vi "AFM_Lithography.vi"() -> ()   [LabVIEW 2019]
uses:
  subVIs/Global Variables.vi
  <vilib>/Analysis/Matrix/Datatypes/RealMatrix.ctl
  <vilib>/Analysis/Matrix/NI_Matrix.lvlib
  <userlib>/LevyLab/Relay Box/Typedefs/Resistor--enum.ctl
  <userlib>/LevyLab/Relay Box/Relay-Box.lvclass
  subVIs/AFM API/AFM_Driver_Manager/AFM_Driver_Manager.lvclass
  <vilib>/vision/Image Controls.llb/IMAQ Image.ctl
  <userlib>/LevyLab/Configuration/Configuration.lvclass
  Controls/Configuration.ctl
  Classes/Parse/ParseVectorFile/ParseVectorFile.lvclass
  <vilib>/JKI/JKI SMO/SMO/SMO.lvclass
  Classes/Settings/Setting Database/Setting Database.lvclass
  Classes/Settings/Setting Database/Typedefs/PrivateEvents--Setting Database.Refresh.ctl
  Classes/Parse/Dot/Dot.lvclass
  Classes/Settings/Dot Settings/Dot Settings.lvclass
  Classes/Settings/Path Settings/Path Settings.lvclass
  Classes/Tool/Tool Data/Tool Data/Tool Data.lvclass
  Classes/Settings/Setting Database/Typedefs/PublicEvents--Setting Database.PathsUpdated.ctl
  Classes/Settings/Rectangle Settings/Rectangle Settings.lvclass
  Classes/Settings/Setting Database/Typedefs/PublicEvents--Setting Database.RectanglesUpdated.ctl
  Classes/Settings/Funnel Settings/Funnel Settings.lvclass
  Classes/Settings/Setting Database/Typedefs/PublicEvents--Setting Database.FunnelsUpdated.ctl
  Classes/Settings/Setting Database/Typedefs/PublicEvents--Setting Database.DotsUpdated.ctl
  Classes/Parse/ParsePaths/Path.lvclass
  Classes/Parse/Rectangle/Rectangle.lvclass
  Classes/Parse/Image/SVGImage.lvclass
  Classes/Tool/Tool Data/Tool Data/Typedefs/PrivateEvents--Tool Data.Update Objects.ctl
  <vilib>/Platform/browser.llb/Open URL in Default Browser (string).vi
  Classes/Selector/Selector.lvclass
  <vilib>/Utility/miscctls.llb/LVPositionTypeDef.ctl
  C:/Program Files (x86)/National Instruments/LabVIEW 2019/vi.lib/JKI/JKI SMO/SMO/SMO.lvclass
  Classes/Settings/ObjectSettings/ObjectSettings.lvclass
  C:/Users/Albro/Documents/GitHub/AFM-Lithography/lvsrc/Classes/Settings/ObjectSettings/ObjectSettings.lvclass
  Classes/Tool/Tool Path/Tool Path.lvclass
  C:/Users/Albro/Documents/GitHub/AFM-Lithography/lvsrc/Classes/Tool/Tool Object/Tool Object.lvclass
  Classes/Tool/Tool Funnel/Tool Funnel.lvclass
  C:/Users/Albro/Documents/GitHub/AFM-Lithography/lvsrc/Classes/Tool/Tool Path/Tool Path.lvclass
  Classes/Tool/Tool Rectangle/Tool Rectangle.lvclass
  Classes/Tool/Tool Dot/Tool Dots.lvclass
panel:
  in  "Listbox":i32(listbox)
  out "version":string
  out "Ready?":bool
  out "Estimated Time":string
  in  "Run":bool
  in  "Refresh Button":bool
  in  "Done":bool
  in  "Help":bool
  in  "Abort":bool
  out "Render":T1(plugin-control)
  in  "Settings":T2(tab)
  out "Status":string
  in  "Background Image":path caption="Path"
  in  "Inkscape File (.svg)":path caption="Path"
  in  "Hide Labels?":bool
  in  "Patterns":i32(listbox) caption="Patterns (drag-and-drop reorder)"
  in  "AFM Type":u16(ring) caption="Ring" items=["Asylum"]
  in  "Save Render":bool caption="Save"
  in  "Autosave?":bool
  in  "Autosave Path":path caption="Path"
  in  "Create Overlay":bool
  out "Image Filename":string
  in  "Image Data Range":cluster{dbl, dbl}(slide)={100.0, 0.0} scale=0.0..100.0
  in  "Page":u32 caption="Numeric" max=3
  in  "MCLB":i32(listbox) caption="Multicolumn Listbox 2"
  # "AFM Lithography"
  # "Render"
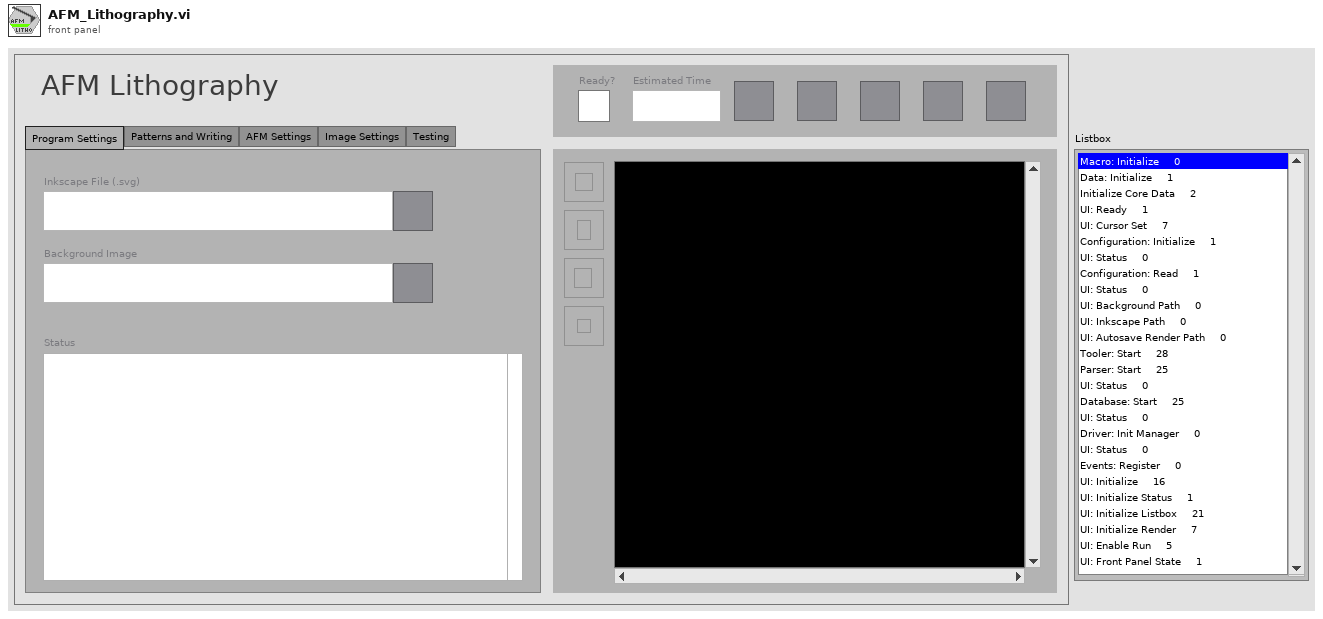
[diagram p1: front panel]
types:
  T1 = typedef "IMAQ Image.ctl" = refnum<image>
  T2 = enum32{"Program Settings", "Patterns and Writing", "AFM Settings", "Image Settings", "Testing"}
  T3 = typedef "LVPositionTypeDef.ctl" = cluster{"Left":i32, "Top":i32}
  T4 = cluster{"Point":T3, "Button":u16, "PlatMods":cluster{"Shift":bool, "Ctrl":bool, "Alt":bool, "Cmd":bool, "Opt":bool}}
  T5 = enum32{"invalid app kind", "Development System", "Run Time System", "Student Edition", "Embedded LabVIEW", "Evaluation", "Custom"}
  T6 = enum32{"Program Settings", "Patterns and Writing", "AFM Settings", "Image Settings"}
  T7 = enum32{"Invalid", "Standard", "Closed", "Hidden", "Minimized", "Maximized"}
  T8 = enum8{"Enabled", "Disabled", "Disabled and Grayed Out"}
  T9 = cluster{"Pattern":string, "Pattern Label":string, "Prompt":string}
  T10 = cluster{"Name":string, "Group":string, "Enabled":bool}
  T11 = typedef "Configuration.ctl" = cluster{"Inkscape Path":path, "Background Path":path, "Autosave Render Path":path, "Autosave Render":bool}
  T12 = typedef "Setting Database.lvclass/PrivateEvents--Setting Database.Refresh.ctl" = cluster{"Paths":string[], "Rectangles":string[], "Funnels":string[], "Dots":string[]}
  T13 = typedef "Tool Data.lvclass/PrivateEvents--Tool Data.Update Objects.ctl" = cluster{"Settings":cluster{"Paths":T14, "Rectangles":T15, "Funnels":T16, "Dots":T17}, "Data":cluster{"Paths":refnum<class "Path.lvclass">[], "Rectangles":refnum<class "Rectangle.lvclass">[], "SVGImage":refnum<class "SVGImage.lvclass">, "Dots":refnum<class "Dot.lvclass">[], "Funnels":refnum<class "Path.lvclass">[]}}
  T14 = typedef "Setting Database.lvclass/PublicEvents--Setting Database.PathsUpdated.ctl" = refnum<class "Path Settings.lvclass">[]
  T15 = typedef "Setting Database.lvclass/PublicEvents--Setting Database.RectanglesUpdated.ctl" = refnum<class "Rectangle Settings.lvclass">[]
  T16 = typedef "Setting Database.lvclass/PublicEvents--Setting Database.FunnelsUpdated.ctl" = refnum<class "Funnel Settings.lvclass">[]
  T17 = typedef "Setting Database.lvclass/PublicEvents--Setting Database.DotsUpdated.ctl" = refnum<class "Dot Settings.lvclass">[]
  T18 = typedef "NI_Matrix.lvlib/RealMatrix.ctl" = dbl[][]
  T19 = typedef "Relay-Box.lvclass/Resistor--enum.ctl" = enum16{"open", "discharge tip", "0 ohms", "100k ohm", "10M ohm", "1G ohm"}
  T20 = cluster{"Core":cluster{"Current VI Reference":refnum<vi>, "Close Panel on Exit?":bool}, "Parsing Data":cluster{"paths":cluster{"Fill Color":string, "Stroke Color":string, "Commands":cluster{"Command Type":string, "Coordinates":cluster{"X":dbl, "Y":dbl}[]}[], "Transformation Matrix 2":T18}[], "funnels":cluster{"Fill Color":string, "Stroke Color":string, "Commands":cluster{"Command Type":string, "Coordinates":cluster{"X":dbl, "Y":dbl}[]}[], "Transformation Matrix 2":T18}[], "rects":cluster{"Fill Color":string, "Stroke Color":string, "Width":dbl, "Height":dbl, "X":dbl, "Y":dbl, "Transformation Matrix":T18}[], "Dots":refnum<class "Dot.lvclass">[]}, "Lithography Data":cluster{"Name":string, "Litho":cluster{"X":dbl, "Y":dbl, "Speed":dbl, "Voltage":dbl}[], "Set Resistance":T19, "Meta":variant}[], "VI Refs":refnum<vi>[], "root path":path, "AFM_Driver_Manager":refnum<class "AFM_Driver_Manager.lvclass">, "IMAQ (Work)":T1, "Background Image":path, "Inkscape File (.svg)":path, "ParseVectorFile":refnum<class "ParseVectorFile.lvclass">, "Database":refnum<class "Setting Database.lvclass">, "Hide Labels":bool, "Autosave?":bool, "Autosave Path":path, "Image Data Range":cluster{dbl, dbl}, "Status":string, "Config":refnum<class "Configuration.lvclass">, "Drag and Drop":cluster{"Start":string[], "End":string[], "Running":string[], "Working":string[]}, "IDs":cluster{"paths":string[], "funnels":string[], "rects":string[], "dots":string[]}, "Tooler":refnum<class "Tool Data.lvclass">, "MCLB":refnum<class "Selector.lvclass">, "Menu Path":string, "Item Names":string[][]}
  T21 = cluster{"Paths":T14, "Rectangles":T15, "Funnels":T16, "Dots":T17}
  T22 = typedef "LVPoint32TypeDef.ctl" = cluster{"Horizontal":i32, "Vertical":i32}
  T23 = cluster{"Shift":bool, "Ctrl":bool, "Alt":bool, "Cmd":bool, "Opt":bool}
  T24 = cluster{"paths":string[], "funnels":string[], "rects":string[], "dots":string[]}
  T25 = cluster{"Start":string[], "End":string[], "Running":string[], "Working":string[]}
  T26 = cluster{"paths":cluster{"Fill Color":string, "Stroke Color":string, "Commands":cluster{"Command Type":string, "Coordinates":cluster{"X":dbl, "Y":dbl}[]}[], "Transformation Matrix 2":T18}[], "funnels":cluster{"Fill Color":string, "Stroke Color":string, "Commands":cluster{"Command Type":string, "Coordinates":cluster{"X":dbl, "Y":dbl}[]}[], "Transformation Matrix 2":T18}[], "rects":cluster{"Fill Color":string, "Stroke Color":string, "Width":dbl, "Height":dbl, "X":dbl, "Y":dbl, "Transformation Matrix":T18}[], "Dots":refnum<class "Dot.lvclass">[]}
  T27 = cluster{"Name":string, "Litho":cluster{"X":dbl, "Y":dbl, "Speed":dbl, "Voltage":dbl}[], "Set Resistance":T19, "Meta":variant}[]
  T28 = cluster{"Current VI Reference":refnum<vi>, "Close Panel on Exit?":bool}
  T29 = typedef "Setting Database.lvclass/PublicEvents--Cluster.ctl" = cluster{"NewActivePath":refnum<user-event>, "PathsUpdated":refnum<user-event>, "RectanglesUpdated":refnum<user-event>, "NewActiveRectangle":refnum<user-event>, "NewActiveFunnel":refnum<user-event>, "FunnelsUpdated":refnum<user-event>, "NewActiveDot":refnum<user-event>, "DotsUpdated":refnum<user-event>}
  T30 = typedef "AFM_Driver_Manager.lvclass/AFM_Driver_Manager.PublicEvents.ctl" = cluster{"Lithography Done":refnum<user-event>}
  T31 = typedef "Image Type" = u32
  T32 = cluster{"Name":string, "Litho":cluster{"X":dbl, "Y":dbl, "Speed":dbl, "Voltage":dbl}[], "Set Resistance":T19, "Meta":variant}
  T33 = cluster{"Name":string, "Group":string, "Enabled":bool}[]
  T34 = typedef "ParseVectorFile.lvclass/PublicEvents--ParseVectorFile.ParsedData.ctl" = cluster{"Paths":refnum<class "Path.lvclass">[], "Rectangles":refnum<class "Rectangle.lvclass">[], "SVGImage":refnum<class "SVGImage.lvclass">, "Dots":refnum<class "Dot.lvclass">[]}
  T35 = cluster{"Paths":refnum<class "Path.lvclass">[], "Rectangles":refnum<class "Rectangle.lvclass">[], "SVGImage":refnum<class "SVGImage.lvclass">, "Dots":refnum<class "Dot.lvclass">[], "Funnels":refnum<class "Path.lvclass">[]}
  T36 = typedef "Tool Data.lvclass/PublicEvents--Tool Data.Objects Updated.ctl" = cluster{"Paths":refnum<class "Tool Path.lvclass">[], "Funnels":refnum<class "Tool Funnel.lvclass">[], "Rectangles":refnum<class "Tool Rectangle.lvclass">[], "Dots":refnum<class "Tool Dots.lvclass">[]}
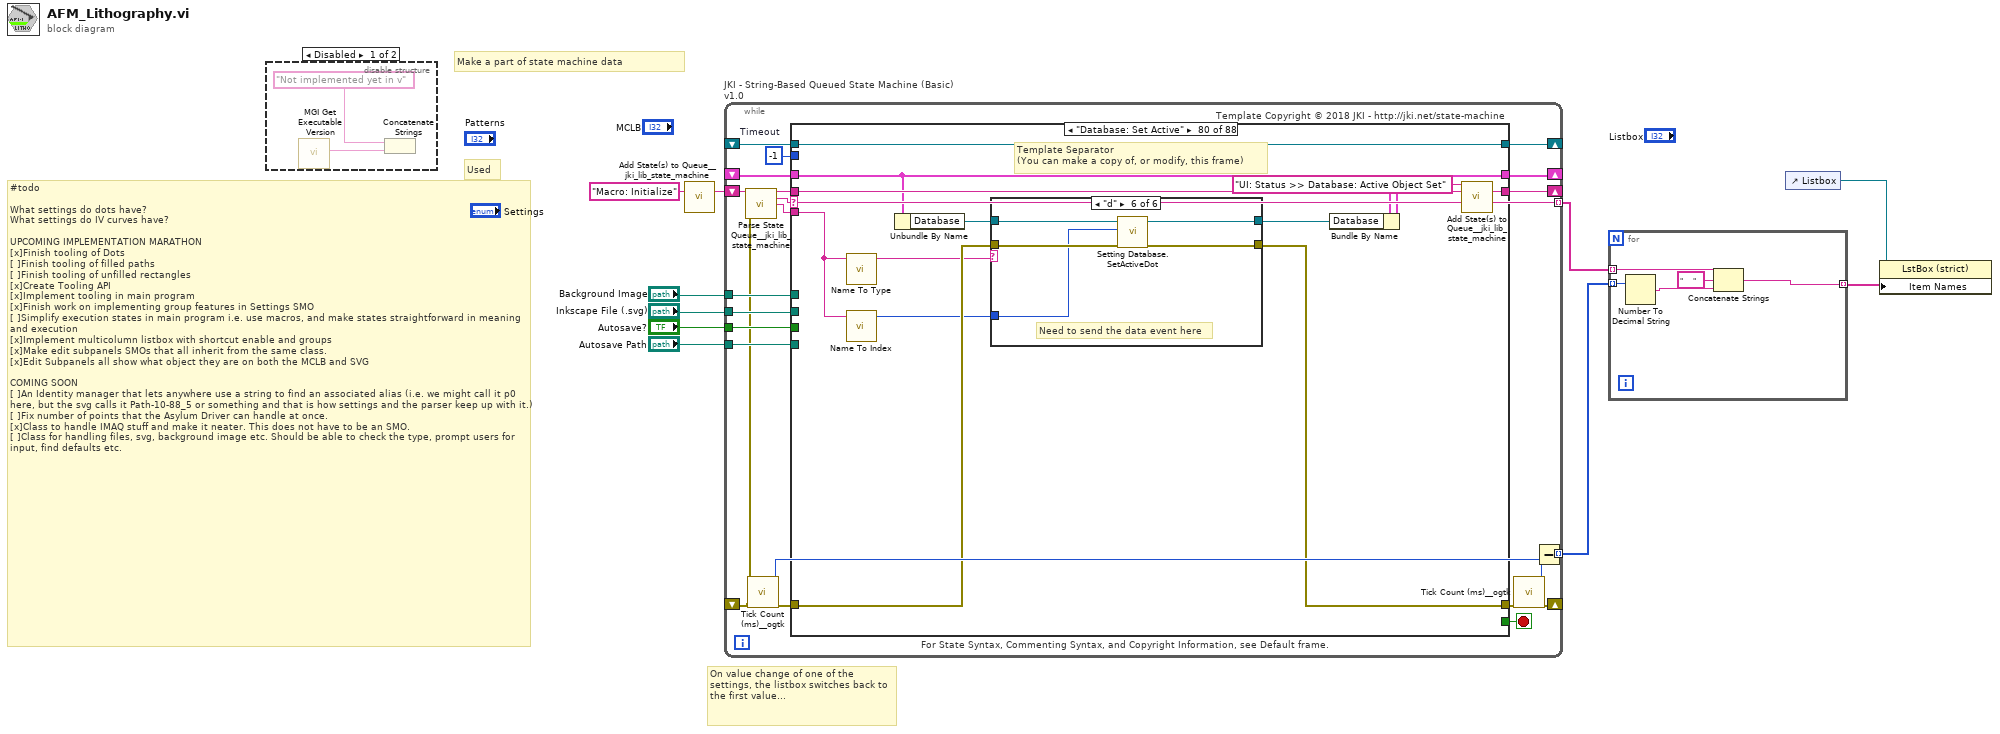
[diagram p0: block diagram]
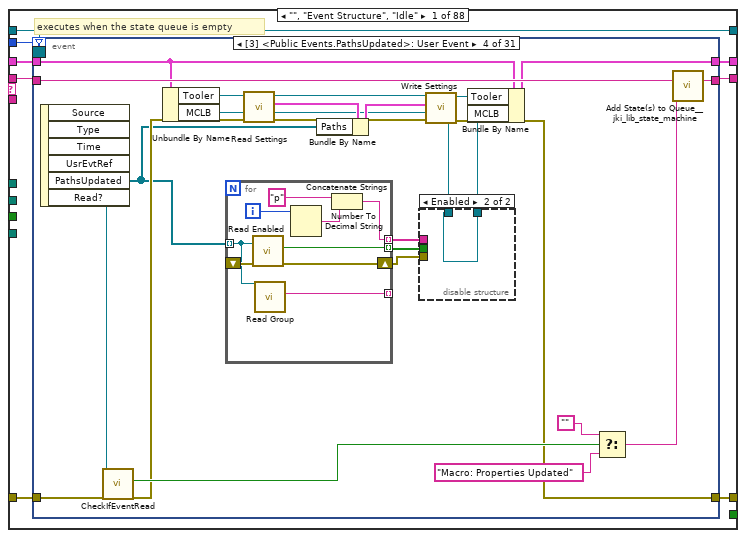
[diagram p3: hidden frame]
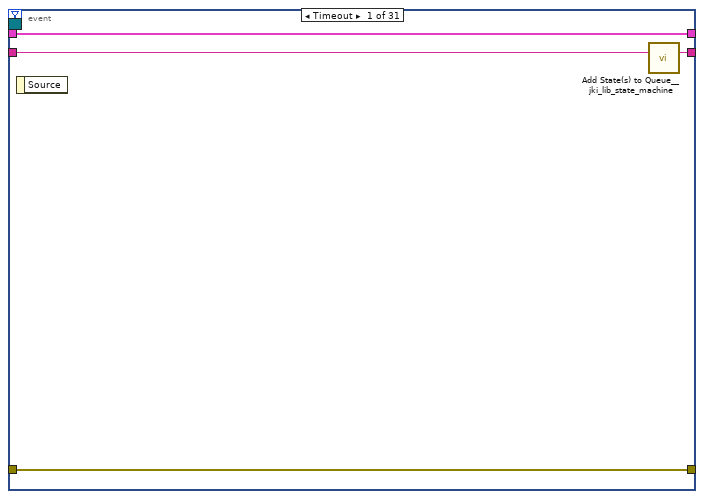
[diagram p4: hidden frame]
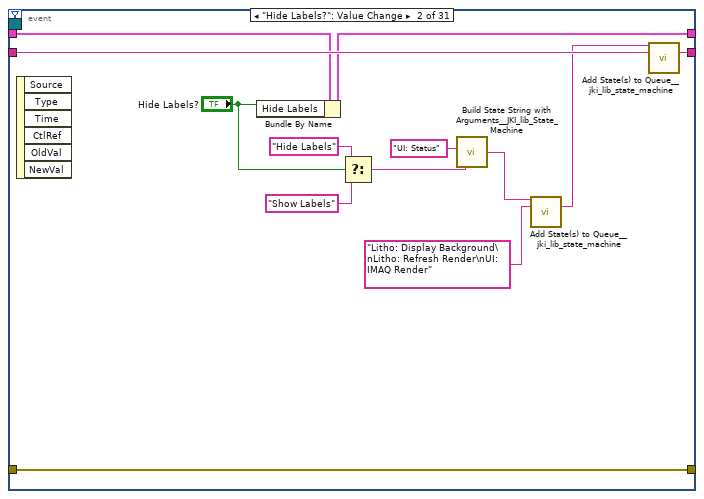
[diagram p5: hidden frame]
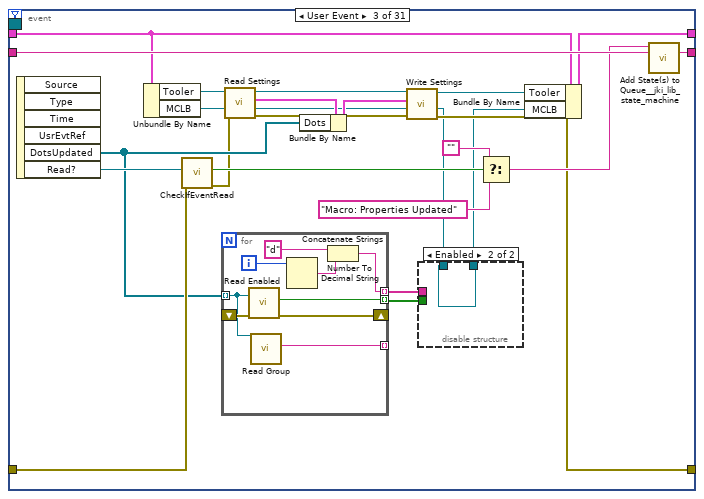
[diagram p6: hidden frame]
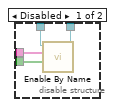
[diagram p7: hidden frame]
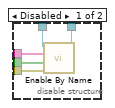
[diagram p8: hidden frame]
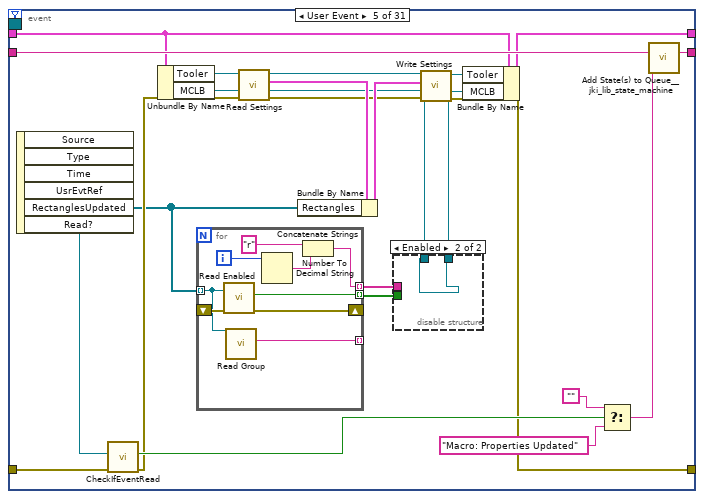
[diagram p9: hidden frame]
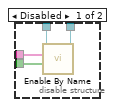
[diagram p10: hidden frame]
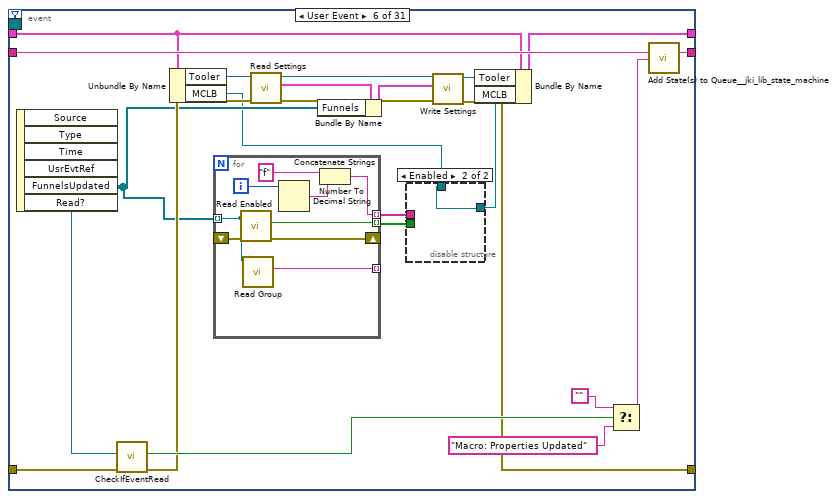
[diagram p11: hidden frame]
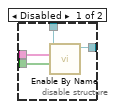
[diagram p12: hidden frame]
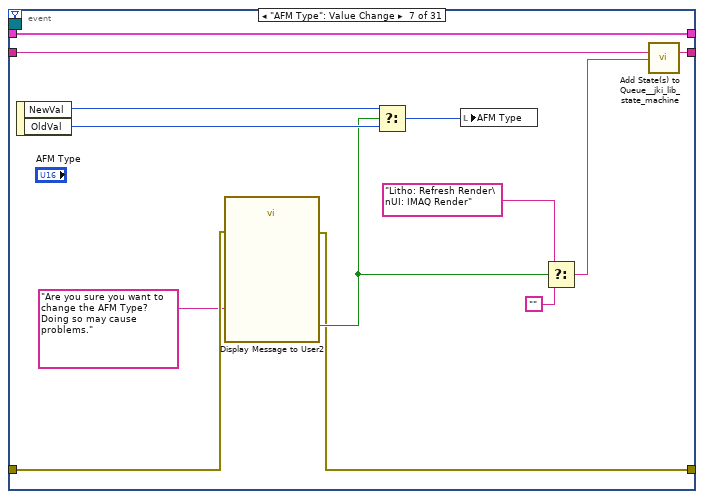
[diagram p13: hidden frame]
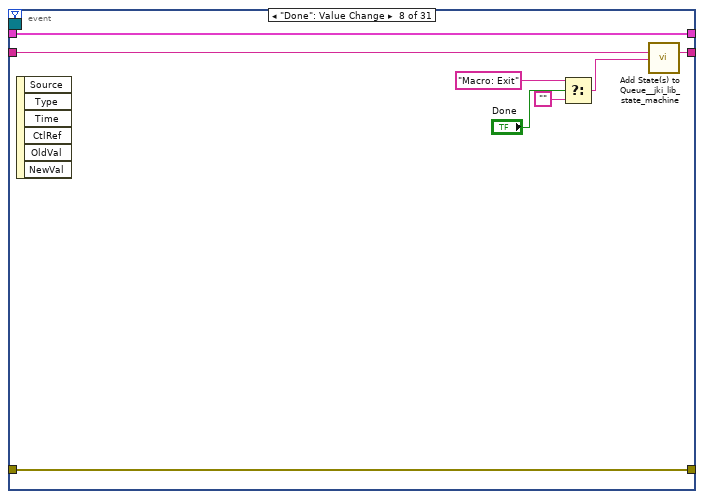
[diagram p14: hidden frame]
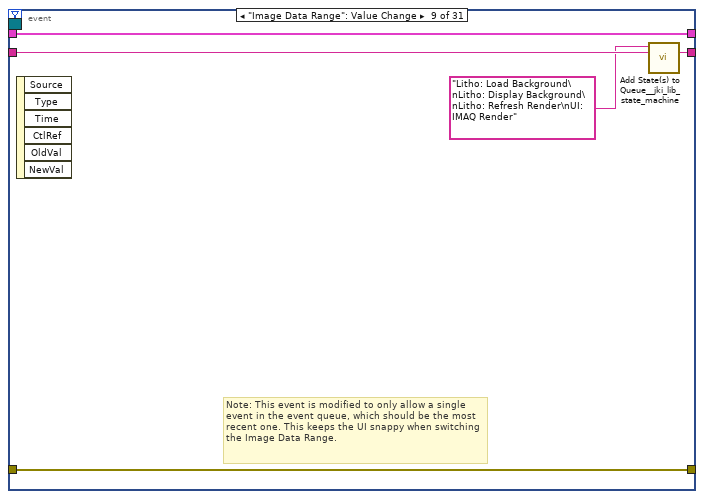
[diagram p15: hidden frame]
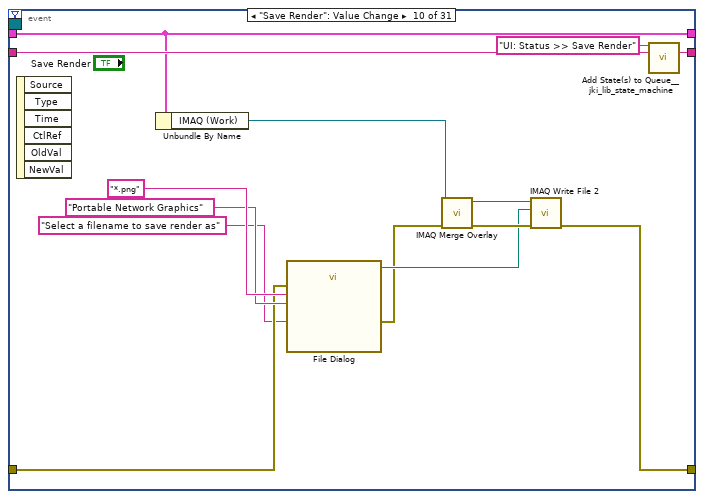
[diagram p16: hidden frame]
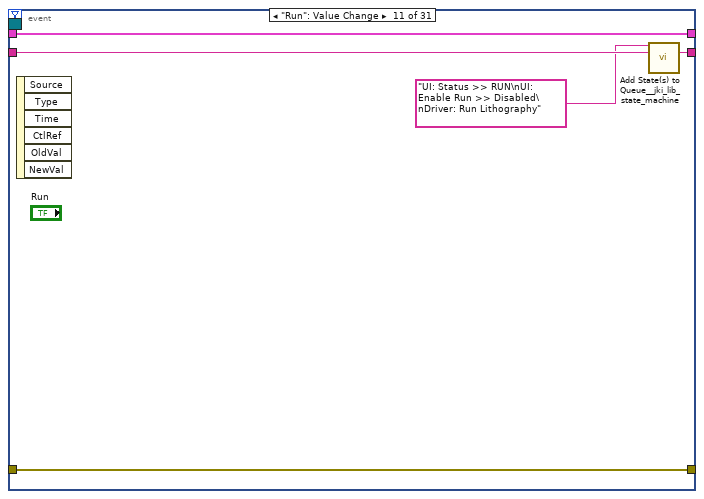
[diagram p17: hidden frame]
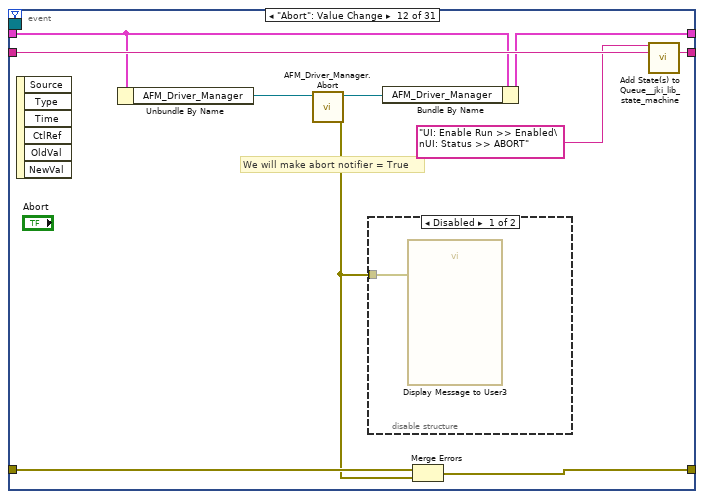
[diagram p18: hidden frame]
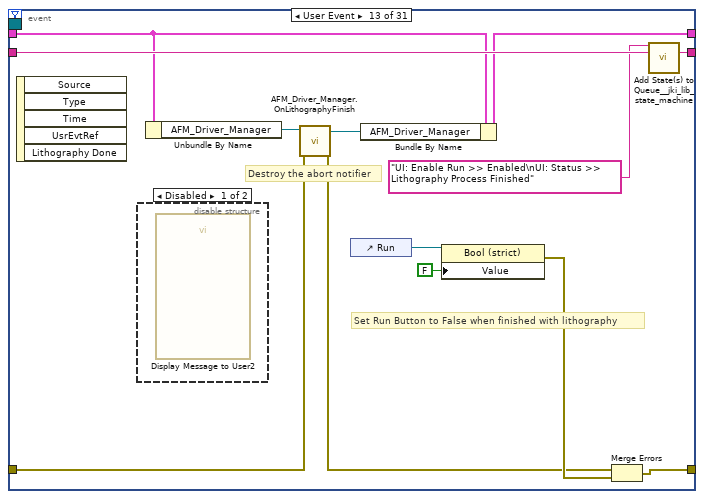
[diagram p20: hidden frame]
diagram:
  # "On value change of one of the settings, the listbox switches back to the first value..."
  # "#todo\n\nWhat settings do dots have?\nWhat settings do IV curves have?\n\nUPCOMING IMPLEMENTATION MARATHON\n[x]Finish tooling of Dots\n[ ]Finish tooling of filled paths\n[ ]Finish tooling of unfilled rectangles\n[x]Create Tooling API\n[x]Implement tooling in main program\n[x]Finish work on implementing group features in Settings SMO\n[ ]Simplify execution states in main program i.e. use macros, and make states straightforward in meaning and execution\n[x]Implement multicolumn listbox with shortcut enable and groups\n[x]Make edit subpanels SMOs that all inherit from the same class.\n[x]Edit Subpanels all show what object they are on both the MCLB and SVG\n\nCOMING SOON\n[ ]An Identity manager that lets anywhere use a string to find an associated alias (i.e. we might call it p0 here, but the svg calls it Path-10-88_5 or something and that is how settings and the parser keep up with it.)\n[ ]Fix number of points that the Asylum Driver can handle at once.\n[x]Class to handle IMAQ stuff and make it neater. This does not have to be an SMO.\n[ ]Class for handling files, svg, background image etc. Should be able to check the type, prompt users for input, find defaults etc."
  # "Used"
  # "Make a part of state machine data"
  n1 = disable-structure shown="Disabled" {
    frame Disabled {
      n2 = call <userlib>:"MGI Get Executable Version.vi"() -> ("Version"=w11:string)  [unwired: 7 in]
      n3 = Concatenate Strings("Not implemented yet in v" ("Status"), w11) -> ()  [unwired: 1 out]
    }
    frame Enabled {
    }
  }
  n4 = call <vilib>:"Add State(s) to Queue__jki_lib_state_machine.vi"("State(s) in (\"\")"="Macro: Initialize") -> ("States Out"=w10:string)  [unwired: 14 in]
  n5 = while "JKI - String-Based Queued State Machine (Basic) v1.0" {
    shift-right: [w32] -> _
    shift-left: _ -> [w31]
    shift-right: [w17] -> _
    shift-left: _ -> [w19]
    shift-right: [w22] -> _
    shift-left: w10 -> [w34]
    shift-right: [w28] -> _
    shift-left: _ -> [w27]
    tunnel: "Background Image" -> [w26]
    tunnel: "Inkscape File (.svg)" -> [w25]
    tunnel: "Autosave?" -> [w24]
    tunnel: "Autosave Path" -> [w23]
    tunnel: [w18] -> w4 mode=indexing
    tunnel: [w13] -> w3 mode=indexing
    stop <- w33 stop-if-true
    w30 = -1  # Timeout
    # "Template Copyright © 2018 JKI - http://jki.net/state-machine"
    # "For State Syntax, Commenting Syntax, and Copyright Information, see Default frame."
    n6 = call <vilib>:"Parse State Queue__jki_lib_state_machine.vi"("State Queue"=w34, "Error In (no error)"=w19) -> ("Remaining States"=w29:string, "Current State"=w18:string, "Arguments"=w21:string)  [unwired: 11 in]
    n7 = call <userlib>:"Tick Count (ms)__ogtk.vi"("error in (no error)"=w19) -> ("error out"=w16:errorcluster, "millisecond timer value"=w14:u32)  [unwired: 9 in]
    n8 = case shown="\"Database: Set Active\"" w18 {
      selector: w18 -> [_ _ w471 _ _ _ _ _ _ _ _ _ _ _ _ _ _ _ _ _ _ _ _ _ _ _ _ _ _ _ _ _ _ _ _ _ _ _ _ _ _ _ _ _ _ _ _ _ _ _ _ _ _ _ _ _ _ _ _ _ _ _ _ _ _ _ _ _ _ _ _ _ _ _ _ _ _ _ _ _ _ _ _ _ _ _ _ _]
      tunnel: w21 -> [_ _ _ _ w498 _ _ _ _ _ _ _ _ _ _ _ _ _ _ w681 w693 w701 w717 w728 _ w771 _ _ _ _ _ _ _ _ _ _ _ _ _ _ _ _ _ _ _ _ _ _ _ _ _ _ _ _ _ _ _ _ _ _ _ _ _ _ _ _ _ w1313 _ _ _ _ _ _ _ _ _ _ w1445 w1455 _ _ _ _ _ _ _ _]
      tunnel: w31 -> [w39 w466 w473 w487 w496 w505 w510 _ w547 w566 w579 w588 w595 w608 w612 w630 w638 w645 w673 w687 w697 w703 w707 w726 w757 w774 w778 w788 w805 w814 w823 w848 w868 w872 w878 w884 w889 w895 w901 w907 w913 w923 w928 w938 w957 w982 w1011 w1021 w1030 w1066 w1076 w1087 w1118 w1126 w1149 w1157 w1171 w1185 w1191 w1214 w1230 w1247 w1265 w1277 w1284 w1288 w1299 w1318 w1329 w1337 w1347 w1357 w1371 w1375 w1408 w1421 w1433 w1439 w1450 w1463 w1510 w1549 w1564 w1576 w1583 w1594 w1605 w1635]
      tunnel: w16 -> [w42 w469 w479 w494 w502 w508 w513 w516 w552 w570 w572 w591 w597 w606 w615 w621 w633 w641 w665 w691 w700 w706 w708 w732 w758 w765 w782 w785 w801 w810 w822 w827 w863 w875 w881 w887 w892 w898 w904 w910 w916 w925 w936 w941 w955 w980 w1014 w1023 w1027 w1056 w1078 w1094 w1113 w1134 w1154 w1156 w1176 w1182 w1196 w1219 w1235 w1239 w1262 w1273 w1286 w1289 w1307 w1315 w1326 w1339 w1344 w1361 w1368 w1380 w1384 w1416 w1427 w1444 w1446 w1460 w1501 w1536 w1555 w1570 w1582 w1588 w1599 w1624]
      tunnel: [w40 w468 w475 w493 w500 w507 w512 w542 w548 w569 w582 w590 w604 w610 w614 w628 w640 w661 w671 w690 w699 w705 w718 w730 w762 w776 w781 w791 w808 w819 w826 w849 w870 w874 w880 w886 w891 w897 w903 w909 w915 w924 w935 w940 w960 w986 w1017 w1022 w1032 w1073 w1077 w1093 w1121 w1133 w1153 w1161 w1175 w1189 w1195 w1218 w1234 w1251 w1269 w1281 w1285 w1296 w1310 w1322 w1333 w1343 w1354 w1365 w1373 w1379 w1413 w1425 w1437 w1443 w1454 w1467 w1514 w1553 w1568 w1580 w1587 w1598 w1609 w1639] -> w22
      tunnel: [_ _ _ _ _ TRUE _ _ _ _ _ _ _ _ _ _ _ _ _ _ _ _ _ _ _ _ _ _ _ _ _ _ _ _ _ _ _ _ _ _ _ _ _ _ _ _ _ _ _ _ _ _ _ _ _ _ _ _ _ _ _ _ _ _ _ _ _ _ _ _ _ _ _ _ _ _ _ _ _ _ _ _ _ _ _ _ _ _] -> w33
      tunnel: [w38 w466 w473 w486 w496 w505 w510 w540 w550 w567 w579 w588 w595 w608 w612 w630 w638 w643 w673 w686 w697 w703 w707 w726 w757 w774 w778 w788 w805 w814 w823 w848 w868 w872 w878 w884 w889 w895 w901 w907 w913 w923 w928 w938 w956 w983 w1015 w1021 w1031 w1067 w1076 w1086 w1118 w1127 w1150 w1158 w1172 w1186 w1192 w1215 w1231 w1248 w1266 w1278 w1284 w1292 w1306 w1320 w1330 w1338 w1349 w1360 w1371 w1376 w1409 w1422 w1434 w1440 w1451 w1464 w1511 w1550 w1565 w1577 w1584 w1595 w1606 w1636] -> w32
      tunnel: w30 -> [w37 _ _ _ _ _ _ _ _ _ _ _ _ _ _ _ _ _ _ _ _ _ _ _ _ _ _ _ _ _ _ _ _ _ _ _ _ _ _ _ _ _ _ _ _ _ _ _ _ _ _ _ _ _ _ _ _ _ _ _ _ _ _ _ _ _ _ _ _ _ _ _ _ _ _ _ _ _ _ _ _ _ _ _ _ _ _ _]
      tunnel: [w41 w469 w480 w494 errorcluster {"status"=FALSE, "code"=0, "source"=""} ("error out") w508 w513 w517 w551 w570 w583 w591 w598 w605 w615 w624 w634 w649 w666 w691 w700 w706 w712 w731 w759 w766 w782 w786 w794 w811 w822 w829 w862 w875 w881 w887 w892 w898 w904 w910 w916 w925 w936 w941 w951 w975 w1007 w1023 w1026 w1055 w1078 w1094 w1112 w1134 w1154 w1156 w1176 w1182 w1196 w1219 w1235 w1238 w1257 w1274 w1286 w1290 w1308 w1316 w1327 w1340 w1345 w1362 w1369 w1380 w1393 w1417 w1428 w1444 w1447 w1461 w1499 w1515 w1557 w1571 w1582 w1589 w1600 w1622] -> w20
      tunnel: w29 -> [w36 w467 w474 w488 w497 w504 w511 w541 w548 w568 w578 w589 w603 w609 w613 w629 w639 w662 w672 w689 w698 w704 w716 w727 w761 w775 w780 w790 w807 w818 w825 w847 w869 w873 w879 w885 w890 w896 w902 w908 w914 w922 w927 w939 w959 w985 w1016 w1020 w1024 w1071 w1075 w1092 w1120 w1132 w1152 w1160 w1174 w1188 w1194 w1217 w1233 w1250 w1268 w1280 w1283 w1295 w1309 w1321 w1332 w1342 w1353 w1364 w1372 w1378 w1412 w1424 w1436 w1442 w1453 w1466 w1513 w1552 w1567 w1579 w1586 w1597 w1608 w1638]
      tunnel: [w35 w465 w470 w482 w495 w503 w509 w539 w544 w563 w575 w587 w602 w607 w611 w627 w637 w652 w667 w688 w696 w702 w715 w725 w760 w773 w779 w789 w806 w817 w824 w846 w864 w871 w877 w882 w888 w894 w900 w906 w912 w918 w926 w937 w958 w984 w1006 w1019 w1029 w1070 w1074 w1091 w1119 w1131 w1151 w1159 w1173 w1187 w1193 w1216 w1232 w1249 w1267 w1279 w1282 w1294 w1301 w1314 w1324 w1335 w1348 w1358 w1367 w1377 w1411 w1423 w1435 w1441 w1452 w1465 w1512 w1551 w1566 w1578 w1585 w1596 w1607 w1637] -> w28
      tunnel: w27 -> [w35 w465 w470 w482 w495 w503 w509 w539 w544 w563 w575 w587 _ w607 w611 w627 w637 w652 w667 w688 w696 w702 w715 w725 w760 w773 w779 w789 w806 w817 w824 w846 w864 w871 w877 w882 w888 w894 w900 w906 w912 w918 w926 w937 w958 w984 w1006 w1019 w1029 w1070 w1074 w1091 w1119 w1131 w1151 w1159 w1173 w1187 w1193 w1216 w1232 w1249 w1267 w1279 w1282 w1294 w1301 w1314 w1324 w1335 w1348 w1358 w1367 w1377 w1411 w1423 w1435 w1441 w1452 w1465 w1512 w1551 w1566 w1578 w1585 w1596 w1607 w1637]
      tunnel: w26 -> [_ _ _ _ _ _ _ w538 _ _ _ _ _ _ _ _ _ _ _ _ _ _ _ _ _ _ _ _ _ _ _ _ _ _ _ _ _ _ _ _ _ _ _ _ _ _ _ _ _ _ _ _ _ _ _ _ _ _ _ _ _ _ _ _ _ _ _ _ _ _ _ _ _ _ _ _ _ _ _ _ _ _ _ _ _ _ _ _]
      tunnel: w25 -> [_ _ _ _ _ _ _ w537 _ _ _ _ _ _ _ _ _ _ _ _ _ _ _ _ _ _ _ _ _ _ _ _ _ _ _ _ _ _ _ _ _ _ _ _ _ _ _ _ _ _ _ _ _ _ _ _ _ _ _ _ _ _ _ _ _ _ _ _ _ _ _ _ _ _ _ _ _ _ _ _ _ _ _ _ _ _ _ _]
      tunnel: w24 -> [_ _ _ _ _ _ _ w527 _ _ _ _ _ _ _ _ _ _ _ _ _ _ _ _ _ _ _ _ _ _ _ _ _ _ _ _ _ _ _ _ _ _ _ _ _ _ _ _ _ _ _ _ _ _ _ _ _ _ _ _ _ _ _ _ _ _ _ _ _ _ _ _ _ _ _ _ _ _ _ _ _ _ _ _ _ _ _ _]
      tunnel: w23 -> [_ _ _ _ _ _ _ w526 _ _ _ _ _ _ _ _ _ _ _ _ _ _ _ _ _ _ _ _ _ _ _ _ _ _ _ _ _ _ _ _ _ _ _ _ _ _ _ _ _ _ _ _ _ _ _ _ _ _ _ _ _ _ _ _ _ _ _ _ _ _ _ _ _ _ _ _ _ _ _ _ _ _ _ _ _ _ _ _]
      frame "", "Event Structure", "Idle" {
        # "executes when the state queue is empty"
        n9 = event shown="[3] <Public Events.PathsUpdated>: User Event" {
          selector: w35 -> [_ _ _ _ _ _ _ _ _ _ _ _ _ _ _ _ _ _ _ _ _ _ _ _ _ _ _ _ _ _ _]
          dyn-events: _ -> [_ _ _ _ _ _ _ _ _ _ _ _ _ _ _ _ _ _ _ _ _ _ _ _ _ _ _ _ _ _ _]
          timeout: w37 -> [_ _ _ _ _ _ _ _ _ _ _ _ _ _ _ _ _ _ _ _ _ _ _ _ _ _ _ _ _ _ _]
          tunnel: w36 -> [w46 w59 w82 w120 w158 w195 w220 w227 w232 w248 w251 w263 w277 w280 w295 w306 w318 w325 w330 w335 w340 w344 w355 w366 w383 w401 w432 w436 w446 w457 w463]
          tunnel: [w45 w58 w81 w119 w157 w194 w221 w228 w233 w249 w252 w264 w278 w281 w294 w305 w317 w324 w329 w334 w339 w343 w354 w365 w382 w400 w431 w435 w445 w456 w462] -> w40
          tunnel: w39 -> [w44 w55 w66 w106 w144 w181 w222 w229 w234 w247 w253 w258 w270 w283 w292 w303 w316 w321 w327 w333 w341 w345 w351 w361 w380 w396 w428 w437 w442 w453 w461]
          tunnel: w42 -> [w43 w57 w76 w118 w154 w191 w212 w230 w235 w239 w254 w260 w271 w285 w296 w307 w319 w326 w331 w336 w337 w346 w347 w357 w384 w390 w433 w438 w440 w458 w464]
          tunnel: [w44 w56 w71 w104 w141 w178 w222 w229 w234 w247 w253 w259 w273 w283 w293 w304 w309 w322 w327 w333 w341 w345 w352 w362 w381 w395 w429 w437 w443 w454 w461] -> w38
          tunnel: [w43 w57 w67 w98 w142 w179 w211 w230 w235 w243 w254 w261 w267 w284 w296 w307 w319 w326 w331 w336 w337 w346 w348 w358 w384 w391 w433 w438 w439 w458 w464] -> w41
          event Timeout {
            n10 = event-data() -> ()  [unwired: 1 in, 1 out]
            n11 = call <vilib>:"Add State(s) to Queue__jki_lib_state_machine.vi"("State(s) in (\"\")"=w46) -> ("States Out"=w45:string)  [unwired: 14 in]
          }
          event "Hide Labels?": Value Change {
            n12 = event-data() -> ()  [unwired: 1 in, 6 out]
            n13 = Bundle By Name(cluster=w55, "Hide Labels"="Hide Labels?") -> (w56:T20)
            n14 = Select(t="Hide Labels" ("State(s) in Front (\"\")"), s="Hide Labels?", f="Show Labels" ("State(s) in Front (\"\")")) -> (s? t:f=w50:string)
            n15 = call <vilib>:"Build State String with Arguments__JKI_lib_State_Machine.vi"("Arguments (\"\")"=w50, "State"="UI: Status") -> ("State with Arguments"=w49:string)  [unwired: 4 in]
            n16 = call <vilib>:"Add State(s) to Queue__jki_lib_state_machine.vi"("State(s) in Front (\"\")"=w49, "State(s) in (\"\")"="Litho: Display Background\nLitho: Refresh Render\nUI: IMAQ Render") -> ("States Out"=w53:string)  [unwired: 13 in]
            n17 = call <vilib>:"Add State(s) to Queue__jki_lib_state_machine.vi"("State(s) in Front (\"\")"=w53, "State(s) in (\"\")"=w59) -> ("States Out"=w58:string)  [unwired: 13 in]
          }
          event User Event {
            n18 = event-data() -> ("DotsUpdated"=w65:T17, "Read?"=w80:refnum<notifier>)  [unwired: 1 in, 4 out]
            n19 = Unbundle By Name(w66) -> ("Tooler"=w74:refnum<class "Tool Data.lvclass">, "MCLB"=w62:refnum<class "Selector.lvclass">)
            n20 = call "CheckIfEventRead.vi"("error in (no error)"=w76, "Read?"=w80) -> ("error out"=w60:errorcluster, "Read"=w75:bool)  [unwired: 8 in]
            n21 = for {
              tunnel: w65 -> [w89] mode=indexing
              tunnel: [w96] -> w63 mode=indexing
              tunnel: [w92] -> w64 mode=indexing
              shift-right: [w91] -> _
              shift-left: _ -> [w90]
              tunnel: [w88] -> _ mode=indexing
              i -> [w94]
              n22 = call "Read Enabled.vi"("error in (no error)"=w90, "ObjectSettings in"=w89) -> ("error out"=w91:errorcluster, "Enabled"=w96:bool)  [unwired: 7 in, 1 out]
              n23 = call-dynamic "Read Group.vi"("ObjectSettings in"=w89) -> ("Group"=w88:string)  [unwired: 8 in, 2 out]
              n24 = Number To Decimal String(number=w94) -> (decimal integer string=w93:string)  [unwired: 1 in]
              n25 = Concatenate Strings("d" ("string"), w93) -> (w92:string)
            }
            n26 = call-dynamic "Read Settings.vi"("error in (no error)"=w60, "Tool Data in"=w74) -> ("error out"=w68:errorcluster, "Settings"=w70:T21, "Tool Data out"=w73:refnum<class "Tool Data.lvclass">)  [unwired: 7 in]
            n27 = Bundle By Name(cluster=w70, "Dots"=w65) -> (w69:T21)
            n28 = call-dynamic "Write Settings.vi"("error in (no error)"=w68, "Settings"=w69, "Tool Data in"=w73) -> ("error out"=w67:errorcluster, "Tool Data out"=w72:refnum<class "Tool Data.lvclass">)  [unwired: 7 in]
            n29 = disable-structure shown="Enabled" {
              disable-tunnel: w64 -> [w86 _]
              disable-tunnel: w63 -> [w85 _]
              disable-tunnel: w62 -> [w84 w87]
              disable-tunnel: [w83 w87] -> w61
              frame Disabled {
                n30 = call-dynamic "Enable By Name.vi"("Enable Items"=w85, "Names"=w86, "Selector in"=w84) -> ("Selector out"=w83:refnum<class "Selector.lvclass">)  [unwired: 7 in, 1 out]
              }
              frame Enabled {
              }
            }
            n31 = Select(t="", s=w75, f="Macro: Properties Updated") -> (s? t:f=w77:string)
            n32 = Bundle By Name(cluster=w66, "Tooler"=w72, "MCLB"=w61) -> (w71:T20)
            n33 = call <vilib>:"Add State(s) to Queue__jki_lib_state_machine.vi"("State(s) in Front (\"\")"=w77, "State(s) in (\"\")"=w82) -> ("States Out"=w81:string)  [unwired: 13 in]
          }
          event User Event {
            n34 = event-data() -> ("PathsUpdated"=w101:T14, "Read?"=w117:refnum<notifier>)  [unwired: 1 in, 4 out]
            n35 = call "CheckIfEventRead.vi"("error in (no error)"=w118, "Read?"=w117) -> ("error out"=w105:errorcluster, "Read"=w113:bool)  [unwired: 8 in]
            n36 = Unbundle By Name(w106) -> ("Tooler"=w112:refnum<class "Tool Data.lvclass">, "MCLB"=w100:refnum<class "Selector.lvclass">)
            n37 = for {
              tunnel: w101 -> [w128] mode=indexing
              tunnel: [w135] -> w102 mode=indexing
              tunnel: [w131] -> w103 mode=indexing
              shift-right: [w130] -> w97
              shift-left: _ -> [w129]
              tunnel: [w127] -> _ mode=indexing
              i -> [w133]
              n38 = call "Read Enabled.vi"("error in (no error)"=w129, "ObjectSettings in"=w128) -> ("error out"=w130:errorcluster, "Enabled"=w135:bool)  [unwired: 7 in, 1 out]
              n39 = call-dynamic "Read Group.vi"("ObjectSettings in"=w128) -> ("Group"=w127:string)  [unwired: 8 in, 2 out]
              n40 = Number To Decimal String(number=w133) -> (decimal integer string=w132:string)  [unwired: 1 in]
              n41 = Concatenate Strings("p" ("string"), w132) -> (w131:string)
            }
            n42 = call-dynamic "Read Settings.vi"("error in (no error)"=w105, "Tool Data in"=w112) -> ("error out"=w107:errorcluster, "Settings"=w109:T21, "Tool Data out"=w111:refnum<class "Tool Data.lvclass">)  [unwired: 7 in]
            n43 = Bundle By Name(cluster=w109, "Paths"=w101) -> (w108:T21)
            n44 = disable-structure shown="Enabled" {
              disable-tunnel: w103 -> [w125 _]
              disable-tunnel: w102 -> [w124 _]
              disable-tunnel: w100 -> [w123 w126]
              disable-tunnel: [w122 w126] -> w99
              disable-tunnel: w97 -> [w121 _]
              frame Disabled {
                n45 = call-dynamic "Enable By Name.vi"("error in (no error)"=w121, "Enable Items"=w124, "Names"=w125, "Selector in"=w123) -> ("Selector out"=w122:refnum<class "Selector.lvclass">)  [unwired: 6 in, 1 out]
              }
              frame Enabled {
              }
            }
            n46 = call-dynamic "Write Settings.vi"("error in (no error)"=w107, "Settings"=w108, "Tool Data in"=w111) -> ("error out"=w98:errorcluster, "Tool Data out"=w110:refnum<class "Tool Data.lvclass">)  [unwired: 7 in]
            n47 = Bundle By Name(cluster=w106, "Tooler"=w110, "MCLB"=w99) -> (w104:T20)
            n48 = Select(t="", s=w113, f="Macro: Properties Updated") -> (s? t:f=w114:string)
            n49 = call <vilib>:"Add State(s) to Queue__jki_lib_state_machine.vi"("State(s) in (\"\")"=w120, "State(s) at Back (\"\")"=w114) -> ("States Out"=w119:string)  [unwired: 13 in]
          }
          event User Event {
            n50 = event-data() -> ("RectanglesUpdated"=w138:T15, "Read?"=w153:refnum<notifier>)  [unwired: 1 in, 4 out]
            n51 = call "CheckIfEventRead.vi"("error in (no error)"=w154, "Read?"=w153) -> ("error out"=w143:errorcluster, "Read"=w151:bool)  [unwired: 8 in]
            n52 = Unbundle By Name(w144) -> ("Tooler"=w150:refnum<class "Tool Data.lvclass">, "MCLB"=w137:refnum<class "Selector.lvclass">)
            n53 = for {
              tunnel: w138 -> [w165] mode=indexing
              tunnel: [w172] -> w139 mode=indexing
              tunnel: [w168] -> w140 mode=indexing
              shift-right: [w167] -> _
              shift-left: _ -> [w166]
              tunnel: [w164] -> _ mode=indexing
              i -> [w170]
              n54 = call "Read Enabled.vi"("error in (no error)"=w166, "ObjectSettings in"=w165) -> ("error out"=w167:errorcluster, "Enabled"=w172:bool)  [unwired: 7 in, 1 out]
              n55 = call-dynamic "Read Group.vi"("ObjectSettings in"=w165) -> ("Group"=w164:string)  [unwired: 8 in, 2 out]
              n56 = Number To Decimal String(number=w170) -> (decimal integer string=w169:string)  [unwired: 1 in]
              n57 = Concatenate Strings("r" ("string"), w169) -> (w168:string)
            }
            n58 = call-dynamic "Read Settings.vi"("error in (no error)"=w143, "Tool Data in"=w150) -> ("error out"=w145:errorcluster, "Settings"=w147:T21, "Tool Data out"=w149:refnum<class "Tool Data.lvclass">)  [unwired: 7 in]
            n59 = Bundle By Name(cluster=w147, "Rectangles"=w138) -> (w146:T21)
            n60 = disable-structure shown="Enabled" {
              disable-tunnel: w140 -> [w162 _]
              disable-tunnel: w139 -> [w161 _]
              disable-tunnel: w137 -> [w160 w163]
              disable-tunnel: [w159 w163] -> w136
              frame Disabled {
                n61 = call-dynamic "Enable By Name.vi"("Enable Items"=w161, "Names"=w162, "Selector in"=w160) -> ("Selector out"=w159:refnum<class "Selector.lvclass">)  [unwired: 7 in, 1 out]
              }
              frame Enabled {
              }
            }
            n62 = call-dynamic "Write Settings.vi"("error in (no error)"=w145, "Settings"=w146, "Tool Data in"=w149) -> ("error out"=w142:errorcluster, "Tool Data out"=w148:refnum<class "Tool Data.lvclass">)  [unwired: 7 in]
            n63 = Bundle By Name(cluster=w144, "Tooler"=w148, "MCLB"=w136) -> (w141:T20)
            n64 = Select(t="", s=w151, f="Macro: Properties Updated") -> (s? t:f=w152:string)
            n65 = call <vilib>:"Add State(s) to Queue__jki_lib_state_machine.vi"("State(s) in (\"\")"=w158, "State(s) at Back (\"\")"=w152) -> ("States Out"=w157:string)  [unwired: 13 in]
          }
          event User Event {
            n66 = event-data() -> ("FunnelsUpdated"=w175:T16, "Read?"=w190:refnum<notifier>)  [unwired: 1 in, 4 out]
            n67 = call "CheckIfEventRead.vi"("error in (no error)"=w191, "Read?"=w190) -> ("error out"=w180:errorcluster, "Read"=w188:bool)  [unwired: 8 in]
            n68 = Unbundle By Name(w181) -> ("Tooler"=w187:refnum<class "Tool Data.lvclass">, "MCLB"=w173:refnum<class "Selector.lvclass">)
            n69 = for {
              tunnel: [w201] -> _ mode=indexing
              tunnel: [w209] -> w176 mode=indexing
              tunnel: [w205] -> w177 mode=indexing
              shift-right: [w204] -> _
              shift-left: _ -> [w203]
              tunnel: [w202] -> _ mode=indexing
              tunnel: w175 -> [w201] mode=indexing
              i -> [w207]
              n70 = call "Read Enabled.vi"("error in (no error)"=w203, "ObjectSettings in"=w201) -> ("error out"=w204:errorcluster, "Enabled"=w209:bool)  [unwired: 7 in, 1 out]
              n71 = call-dynamic "Read Group.vi"("ObjectSettings in"=w201) -> ("Group"=w202:string)  [unwired: 8 in, 2 out]
              n72 = Number To Decimal String(number=w207) -> (decimal integer string=w206:string)  [unwired: 1 in]
              n73 = Concatenate Strings("f" ("string"), w206) -> (w205:string)
            }
            n74 = call-dynamic "Read Settings.vi"("error in (no error)"=w180, "Tool Data in"=w187) -> ("error out"=w182:errorcluster, "Settings"=w184:T21, "Tool Data out"=w186:refnum<class "Tool Data.lvclass">)  [unwired: 7 in]
            n75 = Bundle By Name(cluster=w184, "Funnels"=w175) -> (w183:T21)
            n76 = disable-structure shown="Enabled" {
              disable-tunnel: w177 -> [w199 _]
              disable-tunnel: w176 -> [w198 _]
              disable-tunnel: [w197 w200] -> w174
              disable-tunnel: w173 -> [w196 w200]
              frame Disabled {
                n77 = call-dynamic "Enable By Name.vi"("Enable Items"=w198, "Names"=w199, "Selector in"=w196) -> ("Selector out"=w197:refnum<class "Selector.lvclass">)  [unwired: 7 in, 1 out]
              }
              frame Enabled {
              }
            }
            n78 = call-dynamic "Write Settings.vi"("error in (no error)"=w182, "Settings"=w183, "Tool Data in"=w186) -> ("error out"=w179:errorcluster, "Tool Data out"=w185:refnum<class "Tool Data.lvclass">)  [unwired: 7 in]
            n79 = Bundle By Name(cluster=w181, "Tooler"=w185, "MCLB"=w174) -> (w178:T20)
            n80 = Select(t="", s=w188, f="Macro: Properties Updated") -> (s? t:f=w189:string)
            n81 = call <vilib>:"Add State(s) to Queue__jki_lib_state_machine.vi"("State(s) in (\"\")"=w195, "State(s) at Back (\"\")"=w189) -> ("States Out"=w194:string)  [unwired: 13 in]
          }
          event "AFM Type": Value Change {
            n82 = event-data() -> ("NewVal"=w216:u16, "OldVal"=w215:u16)  [unwired: 1 in]
            n83 = call "Display Message to User2"("error in (no error)"=w212, "Message"="Are you sure you want to change the AFM Type? Doing so may cause problems.") -> ("error out"=w211:errorcluster, "OK?"=w213:bool)  [unwired: 8 in]
            n84 = Select(t=w216, s=w213, f=w215) -> (s? t:f=w214:u16)
            n85 = local write "AFM Type"(w214) -> ()
            n86 = Select(t="Litho: Refresh Render\nUI: IMAQ Render" ("State(s) at Back (\"\")"), s=w213, f="" ("Empty String Constant")) -> (s? t:f=w217:string)
            n87 = call <vilib>:"Add State(s) to Queue__jki_lib_state_machine.vi"("State(s) in (\"\")"=w220, "State(s) at Back (\"\")"=w217) -> ("States Out"=w221:string)  [unwired: 13 in]
          }
          event "Done": Value Change {
            n88 = event-data() -> ()  [unwired: 1 in, 6 out]
            n89 = Select(t="Macro: Exit", s="Done", f="" ("Empty String Constant")) -> (s? t:f=w223:string)
            n90 = call <vilib>:"Add State(s) to Queue__jki_lib_state_machine.vi"("State(s) in (\"\")"=w227, "State(s) at Back (\"\")"=w223) -> ("States Out"=w228:string)  [unwired: 13 in]
          }
          event "Image Data Range": Value Change {
            # "Note: This event is modified to only allow a single event in the event queue, which should be the most recent one. This keeps the UI snappy when switching the Image Data Range."
            n91 = event-data() -> ()  [unwired: 1 in, 6 out]
            n92 = call <vilib>:"Add State(s) to Queue__jki_lib_state_machine.vi"("State(s) in Front (\"\")"="Litho: Load Background\nLitho: Display Background\nLitho: Refresh Render\nUI: IMAQ Render", "State(s) in (\"\")"=w232) -> ("States Out"=w233:string)  [unwired: 13 in]
          }
          event "Save Render": Value Change {
            n93 = event-data() -> ()  [unwired: 1 in, 6 out]
            n94 = Unbundle By Name(w247) -> ("IMAQ (Work)"=w245:T1)
            n95 = call "File Dialog"("prompt"="Select a filename to save render as", "error in"=w239, "pattern (all files)"="*.png", "pattern label"="Portable Network Graphics") -> ("selected path"=w242:path, "error out"=w237:errorcluster)  [unwired: 8 in, 2 out]
            n96 = call "IMAQ Merge Overlay"("error in (no error)"=w237, "Image Src"=w245) -> ("error out"=w246:errorcluster, "Image Dst Out"=w244:T1)  [unwired: 8 in]
            n97 = call-poly "IMAQ Write File 2"("error in (no error)"=w246, "File Path"=w242, "Image"=w244) -> ("error out"=w243:errorcluster)  [unwired: 7 in, 1 out]
            n98 = call <vilib>:"Add State(s) to Queue__jki_lib_state_machine.vi"("State(s) in Front (\"\")"="UI: Status >> Save Render" ("State(s) in Front (\"\")"), "State(s) in (\"\")"=w248) -> ("States Out"=w249:string)  [unwired: 13 in]
          }
          event "Run": Value Change {
            n99 = event-data() -> ()  [unwired: 1 in, 6 out]
            n100 = call <vilib>:"Add State(s) to Queue__jki_lib_state_machine.vi"("State(s) in Front (\"\")"="UI: Status >> RUN\nUI: Enable Run >> Disabled\nDriver: Run Lithography", "State(s) in (\"\")"=w251) -> ("States Out"=w252:string)  [unwired: 13 in]
          }
          event "Abort": Value Change {
            # "We will make abort notifier = True"
            n101 = event-data() -> ()  [unwired: 1 in, 6 out]
            n102 = Unbundle By Name(w258) -> ("AFM_Driver_Manager"=w262:refnum<class "AFM_Driver_Manager.lvclass">)
            n103 = call "AFM_Driver_Manager.Abort.vi"("AFM_Driver_Manager in"=w262) -> ("error out"=w256:errorcluster, "AFM_Driver_Manager out"=w257:refnum<class "AFM_Driver_Manager.lvclass">)  [unwired: 9 in]
            n104 = disable-structure "Diagram Disable Structure" shown="Disabled" {
              disable-tunnel: w256 -> [w265 _]
              frame Disabled {
                n105 = call "Display Message to User3"("error in (no error)"=w265) -> ()  [unwired: 9 in, 2 out]
              }
              frame Enabled {
              }
            }
            n106 = Bundle By Name(cluster=w258, "AFM_Driver_Manager"=w257) -> (w259:T20)
            n107 = Merge Errors(w260, w256) -> (w261:errorcluster)
            n108 = call <vilib>:"Add State(s) to Queue__jki_lib_state_machine.vi"("State(s) in Front (\"\")"="UI: Enable Run >> Enabled\nUI: Status >> ABORT", "State(s) in (\"\")"=w263) -> ("States Out"=w264:string)  [unwired: 13 in]
          }
          event User Event {
            # "Destroy the abort notifier"
            # "Set Run Button to False when finished with lithography"
            n109 = event-data() -> ()  [unwired: 1 in, 5 out]
            n110 = disable-structure "Diagram Disable Structure" shown="Disabled" {
              frame Disabled {
                n111 = call "Display Message to User2"() -> ()  [unwired: 10 in, 2 out]
              }
              frame Enabled {
              }
            }
            n112 = Unbundle By Name(w270) -> ("AFM_Driver_Manager"=w274:refnum<class "AFM_Driver_Manager.lvclass">)
            n113 = call "AFM_Driver_Manager.OnLithographyFinish.vi"("error in (no error)"=w271, "AFM_Driver_Manager in"=w274) -> ("error out"=w268:errorcluster, "AFM_Driver_Manager out"=w272:refnum<class "AFM_Driver_Manager.lvclass">)  [unwired: 8 in]
            n114 = control-ref of="Run"() -> (w276:refnum<vi>)
            n115 = Bundle By Name(cluster=w270, "AFM_Driver_Manager"=w272) -> (w273:T20)
            n116 = property on="Property Node" class="Bool (strict)"(reference=w276, "Value"=FALSE) -> (error out=w269:errorcluster)  [unwired: 1 in, 1 out]
            n117 = Merge Errors(w268, w269) -> (w267:errorcluster)
            n118 = call <vilib>:"Add State(s) to Queue__jki_lib_state_machine.vi"("State(s) in Front (\"\")"="UI: Enable Run >> Enabled\nUI: Status >> Lithography Process Finished" ("State(s) in Front (\"\")"), "State(s) in (\"\")"=w277) -> ("States Out"=w278:string)  [unwired: 13 in]
          }
          event "Help": Value Change {
            n119 = event-data() -> ()  [unwired: 1 in, 6 out]
            n120 = call-poly <vilib>:"Open URL in Default Browser.vi"("error in (no error)"=w285, "URL"="https://github.com/levylabpitt/AFM-Lithography") -> ("error out"=w284:errorcluster)  [unwired: 4 in, 1 out]
            n121 = call <vilib>:"Add State(s) to Queue__jki_lib_state_machine.vi"("State(s) in Front (\"\")"="UI: Status >> HELP" ("State(s) in Front (\"\")"), "State(s) in (\"\")"=w280) -> ("States Out"=w281:string)  [unwired: 13 in]
          }
          event "Inkscape File (.svg)": Value Change {
            n122 = event-data() -> ("NewVal"=w291:path)  [unwired: 1 in, 5 out]
            n123 = Bundle By Name(cluster=w292, "Inkscape File (.svg)"=w291) -> (w293:T20)
            n124 = call <vilib>:"Build State String with Arguments__JKI_lib_State_Machine.vi"("Arguments (\"\")"="Inkscape File Changed" ("Arguments (\"\")"), "State"="UI: Status") -> ("State with Arguments"=w290:string)  [unwired: 4 in]
            n125 = call <vilib>:"Add State(s) to Queue__jki_lib_state_machine.vi"("State(s) in Front (\"\")"=w290, "State(s) in (\"\")"="UI: Ready >> FALSE\nMacro: Refresh\n//Macro: Send Driver\nConfiguration: Write\nUI: Ready >> TRUE") -> ("States Out"=w286:string)  [unwired: 13 in]
            n126 = call <vilib>:"Add State(s) to Queue__jki_lib_state_machine.vi"("State(s) in Front (\"\")"=w286, "State(s) in (\"\")"=w295) -> ("States Out"=w294:string)  [unwired: 13 in]
          }
          event "Autosave?": Value Change {
            n127 = event-data() -> ("NewVal"=w302:bool)  [unwired: 1 in, 5 out]
            n128 = Bundle By Name(cluster=w303, "Autosave?"=w302) -> (w304:T20)
            n129 = Select(t="UI: Autosave Render", s=w302, f="") -> (s? t:f=w301:string)
            n130 = call <vilib>:"Add State(s) to Queue__jki_lib_state_machine.vi"("State(s) in Front (\"\")"="Configuration: Write" ("State(s) in Front (\"\")"), "State(s) in (\"\")"=w301) -> ("States Out"=w297:string)  [unwired: 13 in]
            n131 = call <vilib>:"Add State(s) to Queue__jki_lib_state_machine.vi"("State(s) in Front (\"\")"=w297, "State(s) in (\"\")"=w306) -> ("States Out"=w305:string)  [unwired: 13 in]
          }
          event "Autosave Path": Value Change {
            n132 = event-data() -> ("NewVal"=w315:path)  [unwired: 1 in, 5 out]
            n133 = Bundle By Name(cluster=w316, "Autosave Path"=w315) -> (w309:T20)
            n134 = Unbundle By Name(w309) -> ("Autosave?"=w308:bool)
            n135 = Select(t="UI: Autosave Render", s=w308, f="") -> (s? t:f=w314:string)
            n136 = call <vilib>:"Add State(s) to Queue__jki_lib_state_machine.vi"("State(s) in Front (\"\")"="Configuration: Write" ("State(s) in Front (\"\")"), "State(s) in (\"\")"=w314) -> ("States Out"=w310:string)  [unwired: 13 in]
            n137 = call <vilib>:"Add State(s) to Queue__jki_lib_state_machine.vi"("State(s) in Front (\"\")"=w310, "State(s) in (\"\")"=w318) -> ("States Out"=w317:string)  [unwired: 13 in]
          }
          event "Background Image": Value Change {
            n138 = event-data() -> ("NewVal"=w320:path)  [unwired: 1 in, 5 out]
            n139 = Bundle By Name(cluster=w321, "Background Image"=w320) -> (w322:T20)
            n140 = call <vilib>:"Add State(s) to Queue__jki_lib_state_machine.vi"("State(s) in Front (\"\")"="UI: Status >> Background Image Changed\nUI: Ready >> FALSE\nLitho: Load Background\nLitho: Display Background\nLitho: Refresh Render\nUI: IMAQ Render\nDriver: Background Image\nUI: Ready >> TRUE\nConfiguration: Write", "State(s) in (\"\")"=w325) -> ("States Out"=w324:string)  [unwired: 13 in]
          }
          event "Create Overlay": Value Change {
            n141 = event-data() -> ()  [unwired: 1 in, 6 out]
            n142 = call <vilib>:"Add State(s) to Queue__jki_lib_state_machine.vi"("State(s) in Front (\"\")"="UI: Status >> Create Overlay\nUI: Ready >> FALSE\nUI: Overlay\nUI: Ready >> TRUE", "State(s) in (\"\")"=w330) -> ("States Out"=w329:string)  [unwired: 13 in]
          }
          event "Page": Value Change {
            n143 = event-data() -> ()  [unwired: 1 in, 6 out]
            n144 = call <vilib>:"Add State(s) to Queue__jki_lib_state_machine.vi"("State(s) in Front (\"\")"="UI: Status >> Image Page Changed\nUI: Ready >> FALSE\nLitho: Load Background\nLitho: Display Background\nLitho: Refresh Render\nUI: IMAQ Render\nUI: Ready >> TRUE", "State(s) in (\"\")"=w335) -> ("States Out"=w334:string)  [unwired: 13 in]
          }
          event "Refresh Button": Value Change {
            n145 = event-data() -> ()  [unwired: 1 in, 6 out]
            n146 = call <vilib>:"Add State(s) to Queue__jki_lib_state_machine.vi"("State(s) in Front (\"\")"="UI: Status >> REFRESH\nUI: Ready >> FALSE\nMacro: Refresh\nMacro: Send Driver\nUI: Ready >> TRUE", "State(s) in (\"\")"=w340) -> ("States Out"=w339:string)  [unwired: 13 in]
          }
          event "Patterns": Value Change {
            n147 = event-data() -> ()  [unwired: 1 in, 6 out]
            n148 = call <vilib>:"Add State(s) to Queue__jki_lib_state_machine.vi"("State(s) in (\"\")"=w344, "State(s) at Back (\"\")"="UI: Status >> New Active Object Selected\nUI: Update Subpanel\nLitho: Order Data\nDriver: Litho Data" ("State(s) at Back (\"\")")) -> ("States Out"=w343:string)  [unwired: 13 in]
          }
          event "MCLB": Value Change {
            n149 = event-data() -> ("NewVal"=w349:i32)  [unwired: 1 in, 5 out]
            n150 = Unbundle By Name(w351) -> ("MCLB"=w353:refnum<class "Selector.lvclass">)
            n151 = call-dynamic "Write Value.vi"("error in (no error)"=w347, "Value"=w349, "Selector in"=w353) -> ("error out"=w348:errorcluster, "Selector out"=w350:refnum<class "Selector.lvclass">)  [unwired: 7 in]
            n152 = Bundle By Name(cluster=w351, "MCLB"=w350) -> (w352:T20)
            n153 = call <vilib>:"Add State(s) to Queue__jki_lib_state_machine.vi"("State(s) in (\"\")"=w355) -> ("States Out"=w354:string)  [unwired: 14 in]
          }
          event "MCLB": Shortcut Menu Activation? {
            n154 = event-data() -> ("MenuRef"=w364:refnum<k9>, "Coords"=w363:T22)  [unwired: 1 in, 5 out]
            n155 = Unbundle By Name(w361) -> ("MCLB"=w360:refnum<class "Selector.lvclass">)
            n156 = disable-structure shown="Enabled" {
              disable-tunnel: w364 -> [w372 _]
              disable-tunnel: w363 -> [w371 _]
              disable-tunnel: w360 -> [w370 w374]
              disable-tunnel: [w369 w374] -> w359
              disable-tunnel: [w368 w373] -> w358
              disable-tunnel: w357 -> [w367 w373]
              frame Disabled {
                n157 = call-dynamic "Populate Menu Activation.vi"("error in (no error)"=w367, "Point32"=w371, "MenuRef"=w372, "Selector in"=w370) -> ("error out"=w368:errorcluster, "Selector out"=w369:refnum<class "Selector.lvclass">)  [unwired: 6 in]
              }
              frame Enabled {
              }
            }
            n158 = Bundle By Name(cluster=w361, "MCLB"=w359) -> (w362:T20)
            n159 = event-data("Discard?"=FALSE) -> ()  [unwired: 1 in, 1 out]
            n160 = call <vilib>:"Add State(s) to Queue__jki_lib_state_machine.vi"("State(s) in (\"\")"=w366) -> ("States Out"=w365:string)  [unwired: 14 in]
          }
          event "MCLB": Shortcut Menu Selection (User) {
            n161 = event-data() -> ("ItemPath"=w376:string)  [unwired: 1 in, 7 out]
            n162 = Bundle By Name(cluster=w380, "Menu Path"=w376) -> (w381:T20)
            n163 = Match Pattern(string=w376, regular expression="\\:") -> (before substring=w377:string)  [unwired: 1 in, 3 out]
            n164 = call <vilib>:"Build State String with Arguments__JKI_lib_State_Machine.vi"("Arguments (\"\")"=w377, "State"="MCLB: SCM Selection") -> ("State with Arguments"=w375:string)  [unwired: 4 in]
            n165 = call <vilib>:"Add State(s) to Queue__jki_lib_state_machine.vi"("State(s) in Front (\"\")"=w375, "State(s) in (\"\")"=w383) -> ("States Out"=w382:string)  [unwired: 13 in]
          }
          event "MCLB": Mouse Down? {
            n166 = event-data() -> ("Coords"=w393:T22, "Button"=w392:u16, "PlatMods"=w388:T23)  [unwired: 1 in, 5 out]
            n167 = Unbundle By Name(w396) -> ("MCLB"=w398:refnum<class "Selector.lvclass">)
            n168 = disable-structure shown="Enabled" {
              disable-tunnel: w398 -> [w411 w425]
              disable-tunnel: [w410 w425] -> w397
              disable-tunnel: w393 -> [w409 _]
              disable-tunnel: w392 -> [w408 _]
              disable-tunnel: [w407 w424] -> w391
              disable-tunnel: w390 -> [w406 w424]
              disable-tunnel: [w405 _] -> w389
              disable-tunnel: w388 -> [w404 _]
              disable-tunnel: [w403 _] -> w387
              disable-tunnel: ["Database: Update Enable" _] -> w386
              frame Disabled {
                n169 = Bundle By Name(cluster=T4 {"Point"={"Left"=0, "Top"=0}, "Button"=0, "PlatMods"={"Shift"=FALSE, "Ctrl"=FALSE, "Alt"=FALSE, "Cmd"=FALSE, "Opt"=FALSE}} ("Event Data"), "Point"=w409, "Button"=w408, "PlatMods"=w404) -> (w412:T4)
                n170 = call-dynamic "Handle Mouse Down.vi"("error in (no error)"=w406, "Event Data"=w412, "Selector in"=w411) -> ("error out"=w414:errorcluster, "Enable Change"=w405:bool, "Selector out"=w413:refnum<class "Selector.lvclass">)  [unwired: 6 in]
                n171 = case shown="True" w405 {
                  tunnel: w413 -> [w418 w423]
                  tunnel: w414 -> [w417 w422]
                  tunnel: [w417 w421] -> w407
                  tunnel: [w418 w420] -> w410
                  tunnel: ["" ("Name") w419] -> w403
                  frame False {
                  }
                  frame True {
                    n172 = call "Change Active Enable Symbol.vi"("error in (no error)"=w422, "Selector in"=w423) -> ("error out"=w421:errorcluster, "Name"=w419:string, "Selector out"=w420:refnum<class "Selector.lvclass">)  [unwired: 7 in]
                  }
                }
              }
              frame Enabled {
              }
            }
            n173 = Bundle By Name(cluster=w396, "MCLB"=w397) -> (w395:T20)
            n174 = call <vilib>:"Build State String with Arguments__JKI_lib_State_Machine.vi"("Arguments (\"\")"=w387, "State"=w386) -> ("State with Arguments"=w385:string)  [unwired: 4 in]
            n175 = Select(t=w385, s=w389, f="") -> (s? t:f=w394:string)
            n176 = event-data("Discard?"=w389) -> ()  [unwired: 4 in, 1 out]
            n177 = call <vilib>:"Add State(s) to Queue__jki_lib_state_machine.vi"("State(s) in Front (\"\")"=w394, "State(s) in (\"\")"=w401) -> ("States Out"=w400:string)  [unwired: 13 in]
          }
          event "MCLB": Drag Ended {
            n178 = event-data() -> ("CtlRef"=w430:refnum<vi>)  [unwired: 1 in, 4 out]
            n179 = property class="MCListbox (strict)"(reference=w430) -> ("ItemNames"=w427:string[][])  [unwired: 1 in, 2 out]
            n180 = Bundle By Name(cluster=w428, "Item Names"=w427) -> (w429:T20)
            n181 = call <vilib>:"Add State(s) to Queue__jki_lib_state_machine.vi"("State(s) in Front (\"\")"="MCLB: Reorder", "State(s) in (\"\")"=w432) -> ("States Out"=w431:string)  [unwired: 13 in]
          }
          event "MCLB": Drag Starting {
            n182 = event-data() -> ()  [unwired: 1 in, 10 out]
            n183 = call <vilib>:"Add State(s) to Queue__jki_lib_state_machine.vi"("State(s) in (\"\")"=w436, "State(s) at Back (\"\")"="UI: Status >> New Active Object Selected\nUI: Update Subpanel\nLitho: Order Data\nDriver: Litho Data" ("State(s) at Back (\"\")")) -> ("States Out"=w435:string)  [unwired: 13 in]
          }
          event "Patterns": Drag Starting {
            n184 = event-data() -> ("CtlRef"=w444:refnum<vi>)  [unwired: 1 in, 9 out]
            n185 = property class="LstBox (strict)"(reference=w444, error in=w440) -> (error out=w439:errorcluster, "Item Names"=w441:string[])  [unwired: 1 out]
            n186 = Bundle By Name(cluster=w442, "Drag and Drop.Start"=w441) -> (w443:T20)
            n187 = call <vilib>:"Add State(s) to Queue__jki_lib_state_machine.vi"("State(s) in (\"\")"=w446) -> ("States Out"=w445:string)  [unwired: 14 in]
          }
          event "Patterns": Drag Ended {
            n188 = event-data() -> ("CtlRef"=w455:refnum<vi>)  [unwired: 1 in, 4 out]
            n189 = property class="LstBox (strict)"(reference=w455) -> ("Item Names"=w448:string[])  [unwired: 1 in, 2 out]
            n190 = Unbundle By Name(w453) -> ("Drag and Drop.Start"=w452:string[])
            n191 = Equal?(x=w452, y=w448) -> (x = y?=w451:bool)
            n192 = Select(t="" ("State(s) in Front (\"\")"), s=w451, f="//Listbox: Compare Values\nListbox: Reorder Data\n//Litho: Order Data\nDriver: Litho Data\nLitho: Refresh Render") -> (s? t:f=w447:string)
            n193 = Bundle By Name(cluster=w453, "Drag and Drop.Working"=w448, "Drag and Drop.Running"=w448) -> (w454:T20)
            n194 = call <vilib>:"Add State(s) to Queue__jki_lib_state_machine.vi"("State(s) in Front (\"\")"=w447, "State(s) in (\"\")"=w457) -> ("States Out"=w456:string)  [unwired: 13 in]
          }
          event Panel Close? {
            # "Discard the event because we'll close the front panel ourselves in Macro: Exit"
            # "Close Panel button (pressed) Event\n(this executes Macro: Exit to terminate the VI)"
            n195 = event-data() -> ()  [unwired: 1 in, 1 out]
            n196 = event-data ("Event Filter Node")("Discard?"=TRUE) -> ()  [unwired: 1 in, 1 out]
            n197 = call <vilib>:"Add State(s) to Queue__jki_lib_state_machine.vi"("State(s) in Front (\"\")"="Macro: Exit", "State(s) in (\"\")"=w463) -> ("States Out"=w462:string)  [unwired: 13 in]
          }
        }
      }
      frame "---------- Core ----------" {
        # "Do not put any code in this frame.\n(it is a separator no-op)"
        n198 = call <vilib>:"Add State(s) to Queue__jki_lib_state_machine.vi"("State(s) in (\"\")"=w467) -> ("States Out"=w468:string)  [unwired: 14 in]
      }
      frame Default {
        w477 = 42 items=["No error", "Argument error", "Memory is full", "Out of zone", "End of file", "File already open", "Generic file I/O error", "File not found", "File permission error", "Disk is full", "Duplicate path", "Too many files open", "System feature not enabled", "Resource file not found", "Cannot add resource", "Resource not found", "Image not found", "Image memory error", "Pen does not exist", "Config type invalid", "Config token not found", "Config parse error", "Config memory error", "Bad external code format", "Bad external code offset", "External code not present", "Null window", "Destroy window error", "Null menu", "Print aborted", "Bad print record", "Print driver error", "Windows error during printing", "Memory error during printing", "Print dialog error", "Generic print error", "Invalid device refnum", "Device not found", "Device parameter error", "Device unit error", "Cannot open device", "Device call aborted", "Generic error", "Cancelled by user", "Object ID too low", "Object ID too high", "Object not in heap", "Unknown heap", "Unknown object (invalid DefProc)", "Unknown object (DefProc not in table)", "Message out of range", "Invalid (null) method", "Unknown message", "Manager call not supported", "Bad address", "Network operation in progress", "Network operation timed out", "Connection is busy", "Network attribute not supported", "Network error", "Address in use", "System out of memory", "Connection aborted", "Connection refused", "Not connected", "Already connected", "Connection closed", "Initialization error (interapplication manager)", "Bad occurrence", "Wait on unbound occurrence handler", "Occurrence queue overflow", "Datalog type conflict", "Unused", "Unrecognized type (interapplication manager)", "Memory corrupt", "Failed to make temporary DLL", "Old CIN version", "Drag socket not found", "Failed to load drop-object", "Failed to register OLE object", "Failed to release OLE object", "Format specifier type mismatch", "Unknown format specifier", "Too few format specifiers", "Too many format specifiers", "Scan failed", "Newer CIN version", "Error converting to variant", "Runtime menu error", "Password tampered", "Variant attribute not found", "Incompatible variant data type", "Event data is not available", "Event Store is not present", "Occurrence is not found", "Event Queue is not created", "Event info is not available", "Refnum passed is NULL", "Error retrieving Class GUID", "Error retrieving CoClass GUID", "Error retrieving TypeLib GUID.", "Bad built application magic bytes.", "Specific driver is different from the specific driver associated with the Logical Name.", "There is no session opened to the class driver.", "Max Error", "MAX - Error with config objects", "MAX - Error loading configuration", "MAX - Group not supported"]
        # "State Syntax:\nStateCategory: State >> Argument\nLine Terminator: Line feed\nExample:\nUI: Help >> About\n\nWhere \"UI\" is the state category\nWhere \"Help\" is the state\nWhere \"About\" is the argument\nOther Examples:\nApp Data: Initialize\nUI: Initialize\nHelp >> About\n\nCommenting:\nTo add a comment use \"//\" or \"#\" and all text to the right will be ignored\nCommenting Example:\nUI: Initialize // This initializes the UI\n# This whole line is a comment\n// Another comment line"
        # "For instructions on how to use the JKI State Machine, examples and video tutorials, visit:\nhttp://jki.net/state-machine/\n\nJKI State Machine™\nhttp://jki.net/state-machine/\nCopyright (C) 2005-2018, JKI <info@jki.net>\nALL RIGHTS RESERVED"
        # "Handle mistyped state name (developer tool)"
        # "Current State"
        # "Do not delete, rename, or modify this frame.\n(this is used to capture unhandled states and typos)"
        n199 = Format Into String(format string="Software Exception: Unhandled State \"%s\"." ("message"), error in=w479, w471) -> (resulting string=w476:string, error out=w481:errorcluster)  [unwired: 1 in]
        n200 = call <vilib>:"Error Cluster From Error Code.vi"("show call chain? (False)"=TRUE, "error in (no error)"=w481, "error message (\"\")"=w476, "error code (0)"=w477) -> ("error out"=w480:errorcluster)  [unwired: 5 in]
        n201 = call <vilib>:"Add State(s) to Queue__jki_lib_state_machine.vi"("State(s) in (\"\")"=w474) -> ("States Out"=w475:string)  [unwired: 14 in]
      }
      frame "Initialize Core Data" {
        # "Do not delete, rename, or modify this frame.\n(this is used to determine panel behavior on exit)"
        # "originally closed?"
        # "exe?"
        # "If panel starts closed or is an EXE, then close it when we exit"
        n202 = property on="Property Node" class="VI"() -> ("Front Panel.Open"=w492:bool)  [unwired: 2 in, 2 out]
        n203 = property on="Property Node" class="App"() -> ("App.Kind"=w491:T5)  [unwired: 2 in, 2 out]
        n204 = control-ref of="Current VI Reference"() -> (w489:refnum<vi>)
        n205 = Not(x=w492) -> (.not. x?=w485:bool)
        n206 = Equal?(x=w491, y=T5."Run Time System" ("Application:Kind")) -> (x = y?=w484:bool)
        n207 = Or(x=w485, y=w484) -> (x .or. y?=w490:bool)
        n208 = Bundle By Name(cluster=w487, "Core.Current VI Reference"=w489, "Core.Close Panel on Exit?"=w490) -> (w486:T20)
        n209 = call <vilib>:"Add State(s) to Queue__jki_lib_state_machine.vi"("State(s) in (\"\")"=w488) -> ("States Out"=w493:string)  [unwired: 14 in]
      }
      frame "Error Handler" {
        # "Unhandled Error -- Display it"
        # "Handle any errors here.\nYou can also output any states to clean-up after errors occur"
        # "Clear error"
        n210 = call <vilib>:"General Error Handler.vi"("[error source] (\" \")"=w498, "error in (no error)"=w502) -> ()  [unwired: 9 in, 5 out]
        n211 = call <vilib>:"Add State(s) to Queue__jki_lib_state_machine.vi"("State(s) in Front (\"\")"="/* Post Error States", "State(s) in (\"\")"=w497) -> ("States Out"=w500:string)  [unwired: 13 in]
      }
      frame "Exit" {
        # "Do not put any code in this frame.\n(No errors that occur here will be handled.)"
        n212 = call <vilib>:"Add State(s) to Queue__jki_lib_state_machine.vi"("State(s) in (\"\")"=w504) -> ("States Out"=w507:string)  [unwired: 14 in]
      }
      frame "---------- Data ----------" {
        # "Do not put any code in this frame.\n(It is a separator no-op. You can make a copy of this frame to create a new Data frame)"
        n213 = call <vilib>:"Add State(s) to Queue__jki_lib_state_machine.vi"("State(s) in (\"\")"=w511) -> ("States Out"=w512:string)  [unwired: 14 in]
      }
      frame "Data: Initialize" {
        w514 = string[][] []  # Item Names
        w515 = ""  # Menu Path
        w521 = refnum<class "Tool Data.lvclass"> refnum  # Tooler
        w522 = T24 {"paths"=[], "funnels"=[], "rects"=[], "dots"=[]}  # IDs
        w535 = T25 {"Start"=[], "End"=[], "Running"=[], "Working"=[]}  # Drag and Drop
        w536 = refnum<class "Configuration.lvclass"> refnum  # Config
        w520 = ""  # Status
        w523 = cluster{dbl, dbl} {100.0, 0.0}  # Image Data Range
        w524 = FALSE  # Hide Labels
        w525 = refnum<class "Setting Database.lvclass"> refnum  # Database
        w528 = refnum<class "ParseVectorFile.lvclass"> refnum  # ParseVectorFile
        w529 = T1 refnum  # IMAQ (Work)
        w530 = refnum<class "AFM_Driver_Manager.lvclass"> refnum  # AFM_Driver_Manager
        w531 = path ""  # root path
        w534 = T26 {"paths"=[], "funnels"=[], "rects"=[], "Dots"=[]}  # Parsing Data
        w532 = refnum<vi>[] []  # VI Refs
        w533 = T27 []  # Lithography Data
        w543 = T28 {"Current VI Reference"=refnum, "Close Panel on Exit?"=FALSE}  # Core
        # "Initialize the shift-register data, here.\n(data names are defined by what you wire into the bundle function)"
        n214 = control-ref of="MCLB"() -> (w518:refnum<vi>)
        n215 = call "Constructor.vi"("error in (no error)"=w516, "Reference"=w518) -> ("error out"=w517:errorcluster, "MCLB"=w519:refnum<class "Selector.lvclass">)  [unwired: 8 in]
        n216 = Bundle("Core"=w543, "Parsing Data"=w534, "Lithography Data"=w533, "VI Refs"=w532, "root path"=w531, "AFM_Driver_Manager"=w530, "IMAQ (Work)"=w529, "Background Image"=w538, "Inkscape File (.svg)"=w537, "ParseVectorFile"=w528, "Database"=w525, "Hide Labels"=w524, "Autosave?"=w527, "Autosave Path"=w526, "Image Data Range"=w523, "Status"=w520, "Config"=w536, "Drag and Drop"=w535, "IDs"=w522, "Tooler"=w521, "MCLB"=w519, "Menu Path"=w515, "Item Names"=w514) -> (w540:T20)  [unwired: 1 in]
        n217 = call <vilib>:"Add State(s) to Queue__jki_lib_state_machine.vi"("State(s) in (\"\")"=w541) -> ("States Out"=w542:string)  [unwired: 14 in]
      }
      frame "Data: Run Edit VIs" {
        w545 = path[] [path "subVIs/subpanel/Path Edit.vi", path "subVIs/subpanel/Rect Edit.vi", path "subVIs/subpanel/Funnel Edit.vi", path "subVIs/subpanel/Dot Edit.vi"]  # Edit VIs
        # "#via_ignore Unused Code"
        # "Is this supposed to be unwired?"
        n218 = Unbundle By Name(w547) -> ("root path"=w546:path)
        n219 = for {
          tunnel: w546 -> [w555]
          tunnel: w545 -> [w554] mode=indexing
          tunnel: [w553] -> _ mode=indexing
          n220 = Build Path(base path=w555, name or relative path=w554) -> (appended path=w553:path)
        }
        n221 = for {
          tunnel: [w557] -> w549 mode=indexing
          shift-right: [w560] -> w551
          shift-left: w552 -> [w561]
          tunnel: w545 -> [w556] mode=indexing
          # "Load and run Plugin VIs"
          n222 = Open VI Reference(vi path=w556, error in (no error)=w561) -> (vi reference=w558:refnum<vi>, error out=w562:errorcluster)  [unwired: 4 in]
          n223 = invoke on="Invoke Node" class="VI" method="Run VI"(reference=w558, error in=w562, "Wait until done"=FALSE ("Wait Until Done")) -> (reference out=w557:refnum<vi>, error out=w560:errorcluster)  [unwired: 2 in, 3 out]
        }
        n224 = Bundle By Name(cluster=w547, "VI Refs"=w549) -> (w550:T20)
      }
      frame "Data: Set Root Path" {
        # "For built exes, this will provide the path inside the exe for this VI, and we can use this as a relative path. For unbuilt environments, it provides the path of the VI running it. Since we dont care about this path of this VI, we strip it.\n\nIn other words, this provides a more consistent way to generate relative paths for both exes and development environments."
        # "Do not put any code in this frame.\n(It is a separator no-op. You can make a copy of this frame to create a new Data frame)"
        n225 = call <userlib>:"Current VI's Path__ogtk.vi"() -> ("Current VI's Path (+ Relative)"=w565:path)  [unwired: 1 in]
        n226 = Strip Path(path=w565) -> (stripped path=w564:path)  [unwired: 1 out]
        n227 = Bundle By Name(cluster=w566, "root path"=w564) -> (w567:T20)
        n228 = call <vilib>:"Add State(s) to Queue__jki_lib_state_machine.vi"("State(s) in (\"\")"=w568) -> ("States Out"=w569:string)  [unwired: 14 in]
      }
      frame "Data: Cleanup" {
        # "Cleanup any data and references, here.\n(this is called automatically, by the Macro: Exit)"
        n229 = Unbundle By Name(w579) -> ("Core.Current VI Reference"=w580:refnum<vi>, "VI Refs"=w581:refnum<vi>[], "IMAQ (Work)"=w574:T1)
        n230 = call "IMAQ Dispose"("All Images? (No)"=TRUE, "Image"=w574, "error in (no error)"=w572) -> ("error out"=w571:errorcluster)  [unwired: 3 in]
        n231 = invoke on="AFM Settings" class="SubPnl" method="Remove VI"(error in=w571) -> (error out=w576:errorcluster)  [unwired: 2 in, 2 out]
        n232 = for {
          tunnel: w581 -> [w584] mode=indexing
          shift-right: [w585] -> w577
          shift-left: w576 -> [w586]
          n233 = call "Abort If Not Refnum.vi"("error in (no error)"=w586, "VI in"=w584) -> ("error out"=w585:errorcluster)  [unwired: 9 in]
        }
        n234 = Close Reference(reference=w580, error in (no error)=w577) -> (error out=w583:errorcluster)
        n235 = call <vilib>:"Add State(s) to Queue__jki_lib_state_machine.vi"("State(s) in (\"\")"=w578) -> ("States Out"=w582:string)  [unwired: 14 in]
      }
      frame "---------- Events ----------" {
        # "Do not put any code in this frame.\n(It is a separator no-op. You can make a copy of this frame to create a new UI frame)"
        n236 = call <vilib>:"Add State(s) to Queue__jki_lib_state_machine.vi"("State(s) in (\"\")"=w589) -> ("States Out"=w590:string)  [unwired: 14 in]
      }
      frame "Events: Register" {
        # "Do not put any code in this frame.\n(It is a separator no-op. You can make a copy of this frame to create a new UI frame)"
        n237 = Unbundle By Name(w595) -> ("AFM_Driver_Manager"=w601:refnum<class "AFM_Driver_Manager.lvclass">, "Database"=w594:refnum<class "Setting Database.lvclass">)
        n238 = call "Setting Database.GetPublicEvents.vi"("Setting Database"=w594) -> ("error out"=w592:errorcluster, "Public Events"=w593:T29)  [unwired: 8 in, 1 out]
        n239 = call "AFM_Driver_Manager.GetPublicEvents.vi"("AFM_Driver_Manager in"=w601) -> ("error out"=w596:errorcluster, "AFM_Driver Events"=w600:T30)  [unwired: 8 in, 1 out]
        n240 = register-events(w600, w593) -> (reference out=w602:refnum<event-registration>, error out=w599:errorcluster)  [unwired: 2 in]
        n241 = Merge Errors(w597, w599, w596, w592) -> (w598:errorcluster)
        n242 = call <vilib>:"Add State(s) to Queue__jki_lib_state_machine.vi"("State(s) in (\"\")"=w603) -> ("States Out"=w604:string)  [unwired: 14 in]
      }
      frame "Events: Unregister" {
        # "Do not put any code in this frame.\n(It is a separator no-op. You can make a copy of this frame to create a new UI frame)"
        n243 = Unregister For Events(event registration refnum=w607, error in=w606) -> (error out=w605:errorcluster)
        n244 = call <vilib>:"Add State(s) to Queue__jki_lib_state_machine.vi"("State(s) in (\"\")"=w609) -> ("States Out"=w610:string)  [unwired: 14 in]
      }
      frame "---------- UI ----------" {
        # "Do not put any code in this frame.\n(It is a separator no-op. You can make a copy of this frame to create a new UI frame)"
        n245 = call <vilib>:"Add State(s) to Queue__jki_lib_state_machine.vi"("State(s) in (\"\")"=w613) -> ("States Out"=w614:string)  [unwired: 14 in]
      }
      frame "UI: Initialize" {
        # "Initialize the User Interface, here.\n(this is called automatically, by the Macro: Init)"
        n246 = call <userlib>:"MGI Get Executable Version.vi"() -> ("Version"=w619:string)  [unwired: 7 in]
        n247 = Format Into String(format string="v%s", w619) -> (resulting string=→"version":string)  [unwired: 2 in, 1 out]
        n248 = control-ref of="Image Data Range"() -> (w626:refnum<vi>)
        n249 = disable-structure shown="TARGET_TYPE==RT" {
          frame condition #0 {
            n250 = local write "Settings"(T6."Program Settings" ("Settings")) -> ()
          }
          frame condition #1 (active) {
          }
        }
        n251 = property class="Slide (strict)"(reference=w626, error in=w621, "ShowValTip"=FALSE) -> (error out=w623:errorcluster)  [unwired: 1 out]
        n252 = property on="Hide Labels?" class="Bool (strict)"("Value"=FALSE ("Hide Labels?")) -> ()  [unwired: 2 in, 2 out]
        n253 = call <userlib>:"Fit VI window to Largest Dec__ogtk.vi"("error in (no error)"=w621) -> ("error out"=w622:errorcluster)  [unwired: 5 in, 1 out]
        n254 = Merge Errors(w623, w622) -> (w624:errorcluster)
        n255 = call <vilib>:"Add State(s) to Queue__jki_lib_state_machine.vi"("State(s) in Front (\"\")"="UI: Initialize Status\nUI: Initialize Listbox\nUI: Initialize Render", "State(s) in (\"\")"=w629) -> ("States Out"=w628:string)  [unwired: 13 in]
      }
      frame "UI: Initialize Status" {
        # "Do not put any code in this frame.\n(It is a separator no-op. You can make a copy of this frame to create a new UI frame)"
        n256 = control-ref of="Status"() -> (w636:refnum<vi>)
        n257 = property class="Str"(reference=w636, error in=w633, "Text.FontName"="Consolas" ("Text.Font:Name"), "Text.FontSize"=u32 20 ("Text.Font:Size")) -> (error out=w634:errorcluster)  [unwired: 1 out]
        n258 = call <vilib>:"Add State(s) to Queue__jki_lib_state_machine.vi"("State(s) in (\"\")"=w639) -> ("States Out"=w640:string)  [unwired: 14 in]
      }
      frame "UI: Initialize Listbox" {
        w650 = TRUE ("Drag/Drop:Allow Dragging")
        # "Make listbox look like JKI Flat 2.0"
        # "Initialize the User Interface, here.\n(this is called automatically, by the Macro: Init)"
        n259 = Unbundle By Name(w645) -> ("MCLB"=w642:refnum<class "Selector.lvclass">)
        n260 = control-ref of="Patterns"() -> (w659:refnum<vi>)
        n261 = property on="Property Node" class="LstBox (strict)"(reference=w659, error in=w641, "Active Row"=-2 ("Active Row:Active Row Number"), "Allow Item Drag"=w650, "Allow Drop"=w650, "Top Row"=0) -> (reference out=w648:refnum<vi>, error out=w660:errorcluster, "Item Names"=w646:string[])
        n262 = Bundle By Name(cluster=w645, "Drag and Drop.Running"=w646) -> (w644:T20)
        n263 = property on="Property Node" class="LstBox (strict)"(reference=w648, error in=w660, "CellBG"=u32 16777215 ("Active Row:Cell Background Color"), "CellFontName"="Application Font" ("Font Name"), "CellFontSize"=u32 22 ("Size"), "CellFontColor"=u32 3947580 ("Color"), "SelColor"=u32 11908533 ("Active Row:Cell Background Color")) -> (error out=w653:errorcluster)  [unwired: 1 out]
        n264 = Bundle By Name(cluster=w644, "MCLB"=w642) -> (w643:T20)
        n265 = Merge Errors(w653, w641) -> (w649:errorcluster)
        n266 = call <vilib>:"Add State(s) to Queue__jki_lib_state_machine.vi"("State(s) in (\"\")"=w662) -> ("States Out"=w661:string)  [unwired: 14 in]
      }
      frame "UI: Initialize Render" {
        w669 = FALSE
        w670 = TRUE
        # "Make a JKI Flat UI 2.0 IMAQ control."
        # "Initialize the User Interface, here.\n(this is called automatically, by the Macro: Init)"
        n267 = control-ref of="Render"() -> (w663:refnum<vi>)
        n268 = property on="Property Node" class="ImageControl"(reference=w663, error in=w665, "Annulus Tool Button Visible"=w669, "Closed Freehand Tool Button Visible"=w669, "Ellipse Tool Button Visible"=w669, "Freehand Tool Button Visible"=w669, "Line Tool Button Visible"=w669, "Pan Tool Button Visible"=w670, "Point Tool Button Visible"=w670, "Polygon Tool Button Visible"=w669, "Polyline Tool Button Visible"=w669, "Rectangle Tool Button Visible"=w669, "Rotated Rectangle Tool Button Visible"=w669, "Selection Tool Button Visible"=w670, "Zoom Tool Button Visible"=w670, "Zoom to Fit Mode"=TRUE) -> (error out=w668:errorcluster)  [unwired: 1 out]
        n269 = Merge Errors(w668) -> (w666:errorcluster)
        n270 = call <vilib>:"Add State(s) to Queue__jki_lib_state_machine.vi"("State(s) in (\"\")"=w672) -> ("States Out"=w671:string)  [unwired: 14 in]
      }
      frame "UI: Status" {
        w675 = "\r\n"
        # "Do not put any code in this frame.\n(It is a separator no-op. You can make a copy of this frame to create a new UI frame)"
        n271 = Unbundle By Name(w687) -> ("Status"=w682:string)
        n272 = Format Date/Time String(time format string (%c)="%H:%M:%S --") -> (date/time string=w684:string)  [unwired: 2 in]
        n273 = Concatenate Strings(w684, "\t", w681, w675, w682) -> (w676:string)
        n274 = call <vilib>:"Delimited String to 1D String Array.vi"("delimiter"=w675, "delimited string"=w676) -> ("string array"=w680:string[])  [unwired: 9 in]
        n275 = Array Subset(array=w680, index=0, length=100) -> (w677:string[])
        n276 = call <vilib>:"1D String Array to Delimited String.vi"("delimiter"=w675, "string array"=w677) -> ("delimited string"=w674:string)  [unwired: 9 in]
        "Status" <- w674
        n277 = Bundle By Name(cluster=w687, "Status"=w674) -> (w686:T20)
        n278 = call <vilib>:"Add State(s) to Queue__jki_lib_state_machine.vi"("State(s) in (\"\")"=w689) -> ("States Out"=w690:string)  [unwired: 14 in]
      }
      frame "UI: Ready" {
        # "Do not put any code in this frame.\n(It is a separator no-op. You can make a copy of this frame to create a new UI frame)"
        n279 = Match True/False String(2:"FALSE" ("false string"), 3:"TRUE" ("true string"), 4:w693) -> (0:→"Ready?":bool)  [unwired: 1 out]
        n280 = call <vilib>:"Add State(s) to Queue__jki_lib_state_machine.vi"("State(s) in (\"\")"=w698) -> ("States Out"=w699:string)  [unwired: 14 in]
      }
      frame "UI: Update Time" {
        # "Do not put any code in this frame.\n(It is a separator no-op. You can make a copy of this frame to create a new UI frame)"
        n281 = call <vilib>:"Add State(s) to Queue__jki_lib_state_machine.vi"("State(s) in (\"\")"=w704) -> ("States Out"=w705:string)  [unwired: 14 in]
        "Estimated Time" <- w701
      }
      frame "UI: Cursor Set" {
        # "Argument"
        # "Set and Unset Cursor Busy.\n(Usage: \"UI: Cursor Set >> Busy|Idle\")"
        n282 = Unbundle By Name(w707) -> ("Core.Current VI Reference"=w709:refnum<vi>)
        n283 = call <userlib>:"Tick Count (ms)__ogtk.vi"("error in (no error)"=w708) -> ("error out"=w714:errorcluster, "millisecond timer value"=w710:u32)  [unwired: 9 in]
        n284 = case shown="\"Busy\"" w717 {
          tunnel: w714 -> [w721 w724]
          tunnel: [w720 w723] -> w713
          tunnel: w709 -> [w719 w722]
          frame "Idle", Default {
            n285 = call <vilib>:"Unset Busy.vi"("error in (no error)"=w721, "VI reference (current VI)"=w719) -> ("error out"=w720:errorcluster)  [unwired: 9 in]
          }
          frame "Busy" {
            n286 = call <vilib>:"Set Busy.vi"("error in (no error)"=w724, "VI reference (current VI)"=w722) -> ("error out"=w723:errorcluster)  [unwired: 8 in, 1 out]
          }
        }
        n287 = call <userlib>:"Tick Count (ms)__ogtk.vi"("error in (no error)"=w713) -> ("error out"=w712:errorcluster, "millisecond timer value"=w711:u32)  [unwired: 9 in]
        n288 = Subtract(x=w711, y=w710) -> ()  [unwired: 1 out]
        n289 = call <vilib>:"Add State(s) to Queue__jki_lib_state_machine.vi"("State(s) in (\"\")"=w716) -> ("States Out"=w718:string)  [unwired: 14 in]
      }
      frame "UI: Front Panel State" {
        # "Argument"
        # "Set Front Panel Open or Closed\n(Usage: \"UI: Front Panel State >> Open|Close\")"
        n290 = Unbundle By Name(w726) -> ("Core.Current VI Reference"=w729:refnum<vi>)
        n291 = case shown="\"Open\", Default" w728 {
          tunnel: w732 -> [w737 w749]
          tunnel: [w738 w750] -> w731
          tunnel: w729 -> [w735 w747]
          frame "Open", Default {
            n292 = property on="Property Node" class="VI"(reference=w735, error in=w737) -> (reference out=w734:refnum<vi>, error out=w736:errorcluster, "Front Panel.Open"=w733:bool)
            n293 = case shown="False" w733 {
              tunnel: [w743 w744] -> w738
              tunnel: w736 -> [w742 w744]
              tunnel: w734 -> [w739 _]
              frame False {
                n294 = invoke on="Invoke Node" class="VI" method="FP.Open"(reference=w739, error in=w742, "Activate"=TRUE, "State"=T7."Standard") -> (error out=w743:errorcluster)  [unwired: 1 in, 4 out]
              }
              frame True {
              }
            }
          }
          frame "Close" {
            n295 = property on="Property Node" class="VI"(reference=w747, error in=w749) -> (reference out=w746:refnum<vi>, error out=w748:errorcluster, "Front Panel.Open"=w745:bool)
            n296 = case shown="False" w745 {
              tunnel: [w751 w754] -> w750
              tunnel: w748 -> [w751 w753]
              tunnel: w746 -> [_ w752]
              frame False {
              }
              frame True {
                n297 = invoke on="Invoke Node" class="VI" method="FP.Close"(reference=w752, error in=w753) -> (error out=w754:errorcluster)  [unwired: 1 in, 2 out]
              }
            }
          }
        }
        n298 = call <vilib>:"Add State(s) to Queue__jki_lib_state_machine.vi"("State(s) in (\"\")"=w727) -> ("States Out"=w730:string)  [unwired: 14 in]
      }
      frame "UI: Overlay" {
        # "Do not put any code in this frame.\n(It is a separator no-op. You can make a copy of this frame to create a new UI frame)"
        n299 = Unbundle By Name(w757) -> ("Background Image"=w756:path, "Image Data Range"=w755:cluster{dbl, dbl})
        n300 = call "AFM_OverlayConfigurator.vi"("Error In"=w758, "Image Data Range (Main)"=w755, "Main Image (IBW)"=w756) -> ("Error Out"=w759:errorcluster)  [unwired: 8 in]
        n301 = call <vilib>:"Add State(s) to Queue__jki_lib_state_machine.vi"("State(s) in (\"\")"=w761) -> ("States Out"=w762:string)  [unwired: 14 in]
      }
      frame "UI: Enable Run" {
        # "Do not put any code in this frame.\n(It is a separator no-op. You can make a copy of this frame to create a new UI frame)"
        n302 = Match True/False String(2:"Disabled" ("false string"), 3:"Enabled" ("true string"), 4:w771) -> (0:w770:bool)  [unwired: 1 out]
        n303 = Select(t=T8."Enabled" ("Disabled"), s=w770, f=T8."Disabled and Grayed Out" ("Disabled")) -> (s? t:f=w769:T8)
        n304 = control-ref of="Run"() -> (w772:refnum<vi>)
        n305 = property class="Bool (strict)"(reference=w772, error in=w765, "DisabledEnum"=w769) -> (error out=w766:errorcluster)  [unwired: 1 out]
        n306 = call <vilib>:"Add State(s) to Queue__jki_lib_state_machine.vi"("State(s) in (\"\")"=w775) -> ("States Out"=w776:string)  [unwired: 14 in]
      }
      frame "UI: Inkscape Path" {
        # "Do not put any code in this frame.\n(It is a separator no-op. You can make a copy of this frame to create a new UI frame)"
        n307 = Unbundle By Name(w778) -> ("Inkscape File (.svg)"=w777:path)
        n308 = local write "Inkscape File (.svg)"(w777) -> ()
        n309 = call <vilib>:"Add State(s) to Queue__jki_lib_state_machine.vi"("State(s) in (\"\")"=w780) -> ("States Out"=w781:string)  [unwired: 14 in]
      }
      frame "UI: Background Path" {
        # "Do not put any code in this frame.\n(It is a separator no-op. You can make a copy of this frame to create a new UI frame)"
        n310 = Unbundle By Name(w788) -> ("Background Image"=w784:path)
        n311 = call <vilib>:"Get File Extension.vi"("error in (no error)"=w785, "file"=w784) -> ("error out"=w786:errorcluster, "filename without extension"=→"Image Filename":string, "dup file"=w783:path)  [unwired: 5 in, 2 out]
        n312 = local write "Background Image"(w783) -> ()
        n313 = call <vilib>:"Add State(s) to Queue__jki_lib_state_machine.vi"("State(s) in (\"\")"=w790) -> ("States Out"=w791:string)  [unwired: 14 in]
      }
      frame "UI: IMAQ Render" {
        w800 = T31 4 items=["Grayscale (U8)", "Grayscale (I16)", "Grayscale (SGL)", "Complex (CSG)", "RGB (U32)", "HSL (U32)", "RGB (U64)", "Grayscale (U16)"] ("Image Type")
        # "This removes the flickering when the imaq control was written to since it is by reference. So suppose you had a background image and data already in the control. Then the data gets updated and the user refreshes. It will rewrite the background image, then the new data. So you will have background with data, background, background with data. This creates a flickering effect. If you update the new image on a different reference, and then copy it to the display reference, it will be Image with old data, Image with new data. This does not flicker because there is not the image without data shown at any point."
        # "Do not put any code in this frame.\n(It is a separator no-op. You can make a copy of this frame to create a new UI frame)"
        n314 = call <userlib>:"Tick Count (ms)__ogtk.vi"("error in (no error)"=w801) -> ("error out"=w795:errorcluster, "millisecond timer value"=w792:u32)  [unwired: 9 in]
        n315 = Unbundle By Name(w805) -> ("IMAQ (Work)"=w797:T1)
        n316 = call "Imaq Create"("Image Name"="Render", "Image Type"=w800, "error in (no error)"=w795) -> ("New Image"=w804:T1, "error out"=w799:errorcluster)  [unwired: 2 in]
        n317 = call "IMAQ Copy"("error in (no error)"=w799, "Image Dst"=w804, "Image Src"=w797) -> ("error out"=w798:errorcluster, "Image Dst Out"=→"Render":T1)  [unwired: 3 in]
        n318 = call <userlib>:"Tick Count (ms)__ogtk.vi"("error in (no error)"=w798) -> ("error out"=w794:errorcluster, "millisecond timer value"=w793:u32)  [unwired: 9 in]
        n319 = Subtract(x=w793, y=w792) -> ()  [unwired: 1 out]
        n320 = call <vilib>:"Add State(s) to Queue__jki_lib_state_machine.vi"("State(s) in Front (\"\")"="UI: Status >> IMAQ Rendered" ("State(s) in Front (\"\")"), "State(s) in (\"\")"=w807) -> ("States Out"=w808:string)  [unwired: 13 in]
      }
      frame "UI: Autosave Render" {
        # "Do not put any code in this frame.\n(It is a separator no-op. You can make a copy of this frame to create a new UI frame)"
        n321 = Unbundle By Name(w814) -> ("IMAQ (Work)"=w813:T1, "Autosave Path"=w812:path)
        n322 = call "IMAQ Merge Overlay"("error in (no error)"=w810, "Image Src"=w813) -> ("error out"=w816:errorcluster, "Image Dst Out"=w815:T1)  [unwired: 8 in]
        n323 = call-poly "IMAQ Write File 2"("error in (no error)"=w816, "Image Quality"=u32 512, "File Path"=w812, "Image"=w815) -> ("error out"=w811:errorcluster)  [unwired: 6 in, 1 out]
        n324 = call <vilib>:"Add State(s) to Queue__jki_lib_state_machine.vi"("State(s) in (\"\")"=w818) -> ("States Out"=w819:string)  [unwired: 14 in]
      }
      frame "UI: Autosave Render Path" {
        # "Do not put any code in this frame.\n(It is a separator no-op. You can make a copy of this frame to create a new UI frame)"
        n325 = Unbundle By Name(w823) -> ("Autosave Path"=w821:path, "Autosave?"=w820:bool)
        n326 = local write "Autosave?"(w820) -> ()
        n327 = local write "Autosave Path"(w821) -> ()
        n328 = call <vilib>:"Add State(s) to Queue__jki_lib_state_machine.vi"("State(s) in (\"\")"=w825) -> ("States Out"=w826:string)  [unwired: 14 in]
      }
      frame "UI: Update Subpanel" {
        # "Subpanel is updated to reflect pattern's type."
        n329 = control-ref of="Patterns"() -> (w844:refnum<vi>)
        n330 = Unbundle By Name(w848) -> ("VI Refs"=w828:refnum<vi>[])
        n331 = property class="LstBox (strict)"(reference=w844, error in=w827) -> (error out=w832:errorcluster, "Item Names"=w841:string[], "Value"=w838:i32)  [unwired: 1 out]
        n332 = control-ref of="Properties"() -> (w839:refnum<vi>)
        n333 = Index Array(array=w841, index=w838) -> (element=w833:string)
        n334 = Search/Split String(string=w833, offset (0)=1) -> (substring before match=w840:string)  [unwired: 1 in, 2 out]
        n335 = call <vilib>:"Build State String with Arguments__JKI_lib_State_Machine.vi"("Arguments (\"\")"=w833, "State"="Database: Set Active") -> ("State with Arguments"=w842:string)  [unwired: 4 in]
        n336 = case shown="\"d\"" w840 {
          tunnel: [2 3 0 1] -> w845
          frame "f", Default {
          }
          frame "d" {
          }
          frame "p" {
          }
          frame "r" {
          }
        }
        n337 = property class="SubPnl"(reference=w839, error in=w832) -> (reference out=w834:refnum<vi>, error out=w835:errorcluster, "InsertedVI"=w830:refnum<vi>)
        n338 = Index Array(array=w828, index=w845) -> (element=w831:refnum<vi>)
        n339 = Equal?(x=w831, y=w830) -> (x = y?=w836:bool)
        n340 = case shown="False" w836 {
          tunnel: w835 -> [w854 w856]
          tunnel: [w853 w856] -> w829
          tunnel: w831 -> [w852 _]
          tunnel: w834 -> [w851 _]
          frame False {
            n341 = invoke on="Invoke Node" class="SubPnl" method="Remove VI"(reference=w851, error in=w854) -> (reference out=w850:refnum<vi>, error out=w855:errorcluster)  [unwired: 1 in, 1 out]
            n342 = invoke on="Invoke Node" class="SubPnl" method="Insert VI"(reference=w850, error in=w855, "VI Ref"=w852) -> (error out=w853:errorcluster)  [unwired: 1 in, 3 out]
          }
          frame True {
          }
        }
        n343 = call <vilib>:"Add State(s) to Queue__jki_lib_state_machine.vi"("State(s) in Front (\"\")"=w842, "State(s) in (\"\")"=w847) -> ("States Out"=w849:string)  [unwired: 13 in]
      }
      frame "UI: Update AFM Ring" {
        # "populate AFM Type ring"
        # "Do not put any code in this frame.\n(It is a separator no-op. You can make a copy of this frame to create a new UI frame)"
        n344 = Select(t=string[] ["Asylum"], s=TRUE, f=string[] ["Cypher", "MFP3D", "MFP3D_Lucy", "Simulation"] ("folder names")) -> (s? t:f=w861:string[])
        n345 = property on="AFM Type" class="Ring (strict)"(error in=w863, "Strings []"=w861) -> (error out=w862:errorcluster)  [unwired: 1 in, 1 out]
        n346 = call <vilib>:"Add State(s) to Queue__jki_lib_state_machine.vi"("State(s) in (\"\")"=w869) -> ("States Out"=w870:string)  [unwired: 14 in]
      }
      frame "---------- Macro ----------" {
        # "Do not put any code in this frame.\n(It is a separator no-op. You can make a copy of this frame to create a new Macro frame)"
        n347 = call <vilib>:"Add State(s) to Queue__jki_lib_state_machine.vi"("State(s) in (\"\")"=w873) -> ("States Out"=w874:string)  [unwired: 14 in]
      }
      frame "Macro: Start SMOs" {
        # "Do not put any code in this frame.\n(It is a separator no-op. You can make a copy of this frame to create a new Macro frame)"
        n348 = call <vilib>:"Add State(s) to Queue__jki_lib_state_machine.vi"("State(s) in Front (\"\")"="Parser: Start\nDatabase: Start\nTooler: Start\nDriver: Init Manager", "State(s) in (\"\")"=w879) -> ("States Out"=w880:string)  [unwired: 13 in]
      }
      frame "Macro: Start Driver" {
        # "Do not put any code in this frame.\n(It is a separator no-op. You can make a copy of this frame to create a new Macro frame)"
        n349 = call <vilib>:"Add State(s) to Queue__jki_lib_state_machine.vi"("State(s) in Front (\"\")"="Driver: Init Drivers\nDriver: Set Active\nDriver: Insert Into Subpanel >> 0", "State(s) in (\"\")"=w885) -> ("States Out"=w886:string)  [unwired: 13 in]
      }
      frame "Macro: Reorder" {
        # "Do not put any code in this frame.\n(It is a separator no-op. You can make a copy of this frame to create a new Macro frame)"
        n350 = call <vilib>:"Add State(s) to Queue__jki_lib_state_machine.vi"("State(s) in (\"\")"=w890) -> ("States Out"=w891:string)  [unwired: 14 in]
      }
      frame "Macro: Litho Data" {
        # "Do not put any code in this frame.\n(It is a separator no-op. You can make a copy of this frame to create a new Macro frame)"
        n351 = call <vilib>:"Add State(s) to Queue__jki_lib_state_machine.vi"("State(s) in Front (\"\")"="Litho: Update Information\nListbox: Compare Values\nListbox: Reorder Data\nLitho: Order Data\nDriver: Litho Data\nLitho: Refresh Render" ("State(s) in Front (\"\")"), "State(s) in (\"\")"=w896) -> ("States Out"=w897:string)  [unwired: 13 in]
      }
      frame "Macro: Properties Updated" {
        # "Do not put any code in this frame.\n(It is a separator no-op. You can make a copy of this frame to create a new Macro frame)"
        n352 = call <vilib>:"Add State(s) to Queue__jki_lib_state_machine.vi"("State(s) in Front (\"\")"="//Idle\nUI: Status >> Object Properties Updated\nUI: Ready >> FALSE\nMCLB: Symbols\nMacro: Litho Data\nUI: IMAQ Render\nUI: Ready >> TRUE", "State(s) in (\"\")"=w902) -> ("States Out"=w903:string)  [unwired: 13 in]
      }
      frame "Macro: Send Driver" {
        # "Information that we want to send to the driver all at once. Ie background image and lithography data"
        n353 = call <vilib>:"Add State(s) to Queue__jki_lib_state_machine.vi"("State(s) in Front (\"\")"="Driver: Background Image\nDriver: Litho Data", "State(s) in (\"\")"=w908) -> ("States Out"=w909:string)  [unwired: 13 in]
      }
      frame "Macro: Refresh" {
        # "Do not put any code in this frame.\n(It is a separator no-op. You can make a copy of this frame to create a new Macro frame)"
        n354 = call <vilib>:"Add State(s) to Queue__jki_lib_state_machine.vi"("State(s) in Front (\"\")"="Litho: Load SVG\nParser: Parse SVG\nDatabase: Refresh Sync\nLitho: Load Background\nLitho: Display Background\nMacro: Litho Data\nUI: IMAQ Render", "State(s) in (\"\")"=w914) -> ("States Out"=w915:string)  [unwired: 13 in]
      }
      frame "Macro: Initialize" {
        w919 = FALSE  # debug?
        w921 = "Data: Initialize\nInitialize Core Data\nConfiguration: Initialize\nConfiguration: Read\nEvents: Register\n\nUI: Initialize\nUI: Front Panel State >> Open\n\nData: Set Root Path"  # macro for debugging
        # "On start up:\nData Initialize\nInitialize core data\nPrep the UI\nRead configuration\nStart Subsystems\nRegister for events\nInitialize the UI\nRun the editing VI subpanels\nStart up the AFM driver\nLoad up the SVG\nParse the SVG \nInitialize the database\nRead and display the background image\nTool the data based on default settings\nUpdate and populate the listbox\nUse the listbox to reorder the data\nSend the data to the driver\nRender the overlay on the svg\nCopy the overlay to the IMAQ display"
        # "Initialization Macro\n(This is called once, when the VI starts)"
        n355 = Select(t=w921, s=w919, f="Data: Initialize\nInitialize Core Data\nUI: Ready >> FALSE\nUI: Cursor Set >> Busy\nConfiguration: Initialize\nConfiguration: Read\nMacro: Start SMOs\nEvents: Register\nUI: Initialize\nUI: Enable Run >> Enabled\nUI: Front Panel State >> Open\nData: Set Root Path\nData: Run Edit VIs\nUI: Update AFM Ring\nUI: Update Subpanel\nMacro: Start Driver\nMacro: Refresh\nMacro: Send Driver\nUI: Ready >> TRUE\nUI: Cursor Set >> Idle") -> (s? t:f=w920:string)
        n356 = call <vilib>:"Add State(s) to Queue__jki_lib_state_machine.vi"("State(s) in Front (\"\")"=w920, "State(s) in (\"\")"=w922) -> ("States Out"=w924:string)  [unwired: 13 in]
      }
      frame "Macro: Exit" {
        # "Why is database so far at the end??"
        # "Exit Macro\n(This is called once, when the VI exits)"
        n357 = Unbundle By Name(w928) -> ("Core.Close Panel on Exit?"=w934:bool)
        n358 = Select(t="UI: Front Panel State >> Close", s=w934, f="" ("Empty String Constant")) -> (s? t:f=w931:string)
        n359 = call <vilib>:"Add State(s) to Queue__jki_lib_state_machine.vi"("State(s) in (\"\")"=w931, "State(s) at Back (\"\")"="UI: Enable Run >> Enabled \\\\makes it easier when editing\nParser: Stop\nTooler: Stop\nDriver: Stop Manager\nConfiguration: Write\nData: Cleanup\nEvents: Unregister\nDatabase: Stop\nExit") -> ("States Out"=w929:string)  [unwired: 13 in]
        n360 = call <vilib>:"Add State(s) to Queue__jki_lib_state_machine.vi"("State(s) in Front (\"\")"=w929, "State(s) in (\"\")"=w927) -> ("States Out"=w935:string)  [unwired: 13 in]
      }
      frame "---------- Litho ----------" {
        # "Template Separator\n(You can make a copy of, or modify, this frame)"
        n361 = call <vilib>:"Add State(s) to Queue__jki_lib_state_machine.vi"("State(s) in (\"\")"=w939) -> ("States Out"=w940:string)  [unwired: 14 in]
      }
      frame "Litho: Load SVG" {
        # "Load SVG\nParses the SVG and stores the data obtained from it."
        n362 = Unbundle By Name(w957) -> ("Inkscape File (.svg)"=w954:path)
        n363 = call "CheckFileConformity.vi"("error in (no error)"=w955, "File Data"=T9 {"Pattern"="svg", "Pattern Label"="Scalable Vector Graphics", "Prompt"="Choose an SVG file"}, "Path In"=w954) -> ("error out"=w952:errorcluster, "No File"=w948:bool, "Path Out"=w953:path, "Asked to Change?"=w942:bool)  [unwired: 5 in]
        n364 = case shown="False" w948 {
          tunnel: w953 -> [w962 _]
          tunnel: w952 -> [w961 w965]
          tunnel: [w961 w967] -> w951
          tunnel: [w962 w966] -> w950
          frame False {
          }
          frame True {
            n365 = call "Display Message to User"("error in (no error)"=w965, "Message"="No Valid File Selected. Using Default.") -> ("error out"=w964:errorcluster)  [unwired: 8 in, 1 out]
            n366 = call "GenerateDefaultSVGFile.vi"("error in (no error)"=w964) -> ("error out"=w967:errorcluster, "Path"=w966:path)  [unwired: 9 in]
          }
        }
        n367 = Select(t="", s=w942, f="Configuration: Write") -> (s? t:f=w945:string)
        n368 = call <vilib>:"Add State(s) to Queue__jki_lib_state_machine.vi"("State(s) in Front (\"\")"="UI: Inkscape Path", "State(s) in (\"\")"=w945) -> ("States Out"=w943:string)  [unwired: 13 in]
        n369 = Bundle By Name(cluster=w957, "Inkscape File (.svg)"=w950) -> (w956:T20)
        n370 = call <vilib>:"Add State(s) to Queue__jki_lib_state_machine.vi"("State(s) in Front (\"\")"=w943, "State(s) in (\"\")"=w959) -> ("States Out"=w960:string)  [unwired: 13 in]
      }
      frame "Litho: Load Background" {
        # "Load Background\nLoads the background file into the images."
        n371 = Unbundle By Name(w982) -> ("Background Image"=w981:path)
        n372 = call "CheckFileConformity.vi"("error in (no error)"=w980, "File Data"=T9 {"Pattern"="ibw", "Pattern Label"="Igor Binary Wave", "Prompt"="Choose an IBW file"}, "Path In"=w981) -> ("error out"=w976:errorcluster, "No File"=w968:bool, "Path Out"=w978:path, "Asked to Change?"=w969:bool)  [unwired: 5 in]
        n373 = case shown="True" w968 {
          tunnel: w976 -> [w987 w990]
          tunnel: w978 -> [w988 _]
          tunnel: [w988 w992] -> w977
          tunnel: [w987 w993] -> w975
          frame False {
          }
          frame True {
            n374 = call "Display Message to User3"("error in (no error)"=w990, "Message"="No Valid File Selected. Using Default.") -> ("error out"=w989:errorcluster)  [unwired: 8 in, 1 out]
            n375 = call "GenerateDefaultIBWFile.vi"("error in (no error)"=w989) -> ("error out"=w993:errorcluster, "Path"=w992:path)  [unwired: 9 in]
          }
        }
        n376 = Select(t="", s=w969, f="Configuration: Write") -> (s? t:f=w972:string)
        n377 = Bundle By Name(cluster=w982, "Background Image"=w977) -> (w983:T20)
        n378 = call <vilib>:"Add State(s) to Queue__jki_lib_state_machine.vi"("State(s) in Front (\"\")"="UI: Background Path", "State(s) in (\"\")"=w972) -> ("States Out"=w970:string)  [unwired: 13 in]
        n379 = call <vilib>:"Add State(s) to Queue__jki_lib_state_machine.vi"("State(s) in Front (\"\")"=w970, "State(s) in (\"\")"=w985) -> ("States Out"=w986:string)  [unwired: 13 in]
      }
      frame "Litho: Display Background" {
        # "Added logic so user cannot select a page/image that doesnt exist"
        # "Displays the background from a file"
        n380 = Unbundle By Name(w1011) -> ("Background Image"=w1010:path, "Inkscape File (.svg)"=w1001:path)
        n381 = Unbundle("Image Data Range") -> (w1013:dbl, w1012:dbl)
        n382 = local read "Page"() -> (w1009:u32)
        n383 = Max & Min(x=w1013, y=w1012) -> (max(x,y)=w996:dbl, min(x,y)=w995:dbl)
        n384 = call "Background.vi"("Image data max"=w996, "Image data min"=w995, "error in (no error)"=w1014, "Resolution"=1024, "Page"=w1009, "Image File Path"=w1010) -> ("error out"=w1003:errorcluster, "Max Pages"=w998:i32, "Corrected Page"=w997:i32, "Background out"=w1000:T1)  [unwired: 2 in]
        n385 = control-ref of="Page"() -> (w1008:refnum<vi>)
        n386 = call "SaveBackground.vi"("error in (no error)"=w1003, "Path"=w1001, "Background In"=w1000) -> ("error out"=w1002:errorcluster, "Background Out"=w999:T1)  [unwired: 7 in]
        n387 = property class="DigNum (strict)"(reference=w1008, error in=w1002, "Value"=w997, "Maximum"=w998) -> (error out=w1007:errorcluster)  [unwired: 1 out]
        n388 = Bundle(w996, w995) -> (w994:cluster{dbl, dbl})  [unwired: 1 in]
        n389 = Bundle By Name(cluster=w1011, "Image Data Range"=w994, "IMAQ (Work)"=w999) -> (w1015:T20)
        n390 = call <vilib>:"Add State(s) to Queue__jki_lib_state_machine.vi"("State(s) in (\"\")"=w1016) -> ("States Out"=w1017:string)  [unwired: 14 in]
      }
      frame "Litho: Update Information" {
        # "Update the lithography data (toolpath)\nUses the parsing data and the properties of each pattern to generate the lithography data."
        n391 = call <vilib>:"Add State(s) to Queue__jki_lib_state_machine.vi"("State(s) in Front (\"\")"="Tooler: Objects\nUI: Status >> Settings applied to objects" ("State(s) in Front (\"\")"), "State(s) in (\"\")"=w1020) -> ("States Out"=w1022:string)  [unwired: 13 in]
      }
      frame "Litho: Order Data" {
        n392 = disable-structure shown="Enabled" {
          disable-tunnel: [w1049 w1053] -> w1031
          disable-tunnel: w1030 -> [w1048 w1053]
          disable-tunnel: [w1041 _] -> w1028
          disable-tunnel: w1027 -> [w1039 w1054]
          disable-tunnel: [w1037 w1054] -> w1026
          disable-tunnel: [w1034 _] -> _
          disable-tunnel: [w1033 w1052] -> w1025
          disable-tunnel: w1024 -> [w1033 w1052]
          frame Disabled {
            # "Order the Patterns\nUses the ordering data to fix lithography data."
            n393 = call <userlib>:"Tick Count (ms)__ogtk.vi"("error in (no error)"=w1039) -> ("error out"=w1040:errorcluster, "millisecond timer value"=w1036:u32)  [unwired: 9 in]
            n394 = Unbundle By Name(w1048) -> ("Lithography Data"=w1050:T27)
            n395 = control-ref of="Patterns"() -> (w1047:refnum<vi>)
            n396 = call "Order Patterns.vi"("error in (no error)"=w1040, "Lithography Data"=w1050, "ListBox Reference in"=w1047) -> ("error out"=w1038:errorcluster, "Order Unchanged"=w1042:bool, "Ordered Lithography Data"=w1051:T27)  [unwired: 6 in]
            n397 = Bundle By Name(cluster=w1048, "Lithography Data"=w1051) -> (w1049:T20)
            n398 = call <userlib>:"Tick Count (ms)__ogtk.vi"("error in (no error)"=w1038) -> ("error out"=w1037:errorcluster, "millisecond timer value"=w1035:u32)  [unwired: 9 in]
            n399 = Subtract(x=w1035, y=w1036) -> (x-y=w1034:u32)
            n400 = Select(t="Unchanged Object Order Applied to Data", s=w1042, f="New Object Order Applied to Data" ("Arguments (\"\")")) -> (s? t:f=w1045:string)
            n401 = call <vilib>:"Build State String with Arguments__JKI_lib_State_Machine.vi"("Arguments (\"\")"=w1045, "State"="UI: Status") -> ("State with Arguments"=w1041:string)  [unwired: 4 in]
          }
          frame Enabled {
          }
        }
        n402 = call <vilib>:"Add State(s) to Queue__jki_lib_state_machine.vi"("State(s) in Front (\"\")"=w1028, "State(s) in (\"\")"=w1025) -> ("States Out"=w1032:string)  [unwired: 13 in]
      }
      frame "Litho: Refresh Render" {
        # "Update the images\nUses the lithography data to update the images."
        n403 = Unbundle By Name(w1066) -> ("Lithography Data"=w1072:T27, "IMAQ (Work)"=w1069:T1, "Hide Labels"=w1064:bool, "Autosave?"=w1063:bool)
        n404 = call "Image Generator.vi"("Coerce"=TRUE, "Hide Labels"=w1064, "Lithography Data"=w1072, "error in (no error)"=w1056, "Resolution"=1024, "Image Reference In"=w1069) -> ("error out"=w1055:errorcluster, "Image Reference Out"=w1068:T1)  [unwired: 4 in]
        n405 = Bundle By Name(cluster=w1066, "IMAQ (Work)"=w1068) -> (w1067:T20)
        n406 = Select(t="UI: Autosave Render", s=w1063, f="") -> (s? t:f=w1058:string)
        n407 = call <vilib>:"Add State(s) to Queue__jki_lib_state_machine.vi"("State(s) in Front (\"\")"="UI: Status >> Render Refreshed" ("State(s) in (\"\")"), "State(s) in (\"\")"=w1058) -> ("States Out"=w1060:string)  [unwired: 13 in]
        n408 = call <vilib>:"Add State(s) to Queue__jki_lib_state_machine.vi"("State(s) in Front (\"\")"=w1060, "State(s) in (\"\")"=w1071) -> ("States Out"=w1073:string)  [unwired: 13 in]
      }
      frame "---------- Listbox ----------" {
        # "Template Separator\n(You can make a copy of, or modify, this frame)"
        n409 = call <vilib>:"Add State(s) to Queue__jki_lib_state_machine.vi"("State(s) in (\"\")"=w1075) -> ("States Out"=w1077:string)  [unwired: 14 in]
      }
      frame "Listbox: Compare Values" {
        # "If working is what is al"
        # "Do they have the same"
        # "This should be the only place that we set the running data."
        # "Template Separator\n(You can make a copy of, or modify, this frame)"
        n410 = Unbundle By Name(w1087) -> ("Drag and Drop.Running"=w1085:string[], "Drag and Drop.Working"=w1084:string[])
        n411 = Sort 1D Array(array=w1085) -> (sorted array=w1088:string[])
        n412 = Sort 1D Array(array=w1084) -> (sorted array=w1089:string[])
        n413 = Equal?(x=w1088, y=w1089) -> (x = y?=w1090:bool)
        n414 = case shown="False" w1090 {
          tunnel: w1085 -> [w1095 w1110]
          tunnel: w1084 -> [w1099 _]
          tunnel: [w1100 w1110] -> w1079
          frame False {
            n415 = for {
              tunnel: w1095 -> [w1108]
              tunnel: w1099 -> [w1105] mode=indexing
              tunnel: [w1105] -> w1101 mode=indexing if=w1109
              tunnel: [w1107] -> w1098 mode=indexing if=w1106
              n416 = Search 1D Array(1D array=w1108, element=w1105) -> (index of element=w1107:i32)  [unwired: 1 in]
              n417 = Greater Or Equal To 0?(x=w1107) -> (x >= 0?=w1106:bool)
              n418 = Not(x=w1106) -> (.not. x?=w1109:bool)
            }
            n419 = Sort 1D Array(array=w1098) -> (sorted array=w1097:i32[])
            n420 = for {
              tunnel: w1095 -> [w1104]
              tunnel: w1097 -> [w1103] mode=indexing
              tunnel: [w1102] -> w1096 mode=indexing
              n421 = Index Array(array=w1104, index=w1103) -> (element=w1102:string)
            }
            n422 = Build Array (concatenate)(w1096, w1101) -> (w1100:string[])
          }
          frame True {
          }
        }
        n423 = Equal?(x=w1085, y=w1079) -> (x = y?=w1083:bool)
        n424 = Bundle By Name(cluster=w1087, "Drag and Drop.Running"=w1079) -> (w1086:T20)
        n425 = Select(t="", s=w1083, f="Listbox: Populate") -> (s? t:f=w1080:string)
        n426 = call <vilib>:"Add State(s) to Queue__jki_lib_state_machine.vi"("State(s) in Front (\"\")"=w1080, "State(s) in (\"\")"=w1092) -> ("States Out"=w1093:string)  [unwired: 13 in]
      }
      frame "Listbox: Populate" {
        # "Template Separator\n(You can make a copy of, or modify, this frame)"
        n427 = Unbundle By Name(w1118) -> ("Drag and Drop.Running"=w1114:string[])
        n428 = control-ref of="Patterns"() -> (w1117:refnum<vi>)
        n429 = property class="LstBox (strict)"(reference=w1117, error in=w1113, "Item Names"=w1114, "Value"=0) -> (error out=w1111:errorcluster)  [unwired: 1 out]
        n430 = Merge Errors(w1111) -> (w1112:errorcluster)
        n431 = call <vilib>:"Add State(s) to Queue__jki_lib_state_machine.vi"("State(s) in Front (\"\")"="UI: Update Subpanel", "State(s) in (\"\")"=w1120) -> ("States Out"=w1121:string)  [unwired: 13 in]
      }
      frame "Listbox: Reorder Data" {
        # "Template Separator\n(You can make a copy of, or modify, this frame)"
        n432 = Unbundle By Name(w1126) -> ("Drag and Drop.Running"=w1130:string[], "Lithography Data"=w1129:T27)
        n433 = for {
          shift-right: [w1147] -> w1124
          shift-left: w1130 -> [w1147]
          tunnel: w1129 -> [w1145] mode=indexing
          tunnel: [w1146] -> w1122 mode=indexing
          tunnel: [w1145] -> w1128 mode=indexing
          n434 = Unbundle By Name(w1145) -> ("Name"=w1146:string)
        }
        n435 = Equal?(x=w1124, y=w1122) -> (x = y?=w1123:bool)
        n436 = case shown="False" w1123 {
          tunnel: w1128 -> [w1138 w1144]
          tunnel: [w1137 w1144] -> w1125
          tunnel: w1124 -> [w1136 _]
          tunnel: w1122 -> [w1135 _]
          frame False {
            # "reorder items in lithography"
            n437 = for {
              tunnel: w1135 -> [w1143]
              tunnel: w1136 -> [w1142] mode=indexing
              tunnel: w1138 -> [w1141]
              tunnel: [w1139] -> w1137 mode=indexing
              n438 = Search 1D Array(1D array=w1143, element=w1142) -> (index of element=w1140:i32)  [unwired: 1 in]
              n439 = Index Array(array=w1141, index=w1140) -> (element=w1139:T32)
            }
          }
          frame True {
            # "Order is already correct"
          }
        }
        n440 = Bundle By Name(cluster=w1126, "Lithography Data"=w1125) -> (w1127:T20)
        n441 = call <vilib>:"Add State(s) to Queue__jki_lib_state_machine.vi"("State(s) in (\"\")"=w1132) -> ("States Out"=w1133:string)  [unwired: 14 in]
      }
      frame "---------- MCLB ----------" {
        # "Multicolumn Listbox\n(You can make a copy of, or modify, this frame)"
        n442 = Unbundle By Name(w1149) -> ("MCLB"=w1148:refnum<class "Selector.lvclass">)
        n443 = Bundle By Name(cluster=w1149, "MCLB"=w1148) -> (w1150:T20)
        n444 = call <vilib>:"Add State(s) to Queue__jki_lib_state_machine.vi"("State(s) in (\"\")"=w1152) -> ("States Out"=w1153:string)  [unwired: 14 in]
      }
      frame "MCLB: Symbols" {
        # "Multicolumn Listbox\n(You can make a copy of, or modify, this frame)"
        n445 = Unbundle By Name(w1157) -> ("MCLB"=w1155:refnum<class "Selector.lvclass">)
        n446 = Bundle By Name(cluster=w1157, "MCLB"=w1155) -> (w1158:T20)
        n447 = call <vilib>:"Add State(s) to Queue__jki_lib_state_machine.vi"("State(s) in (\"\")"=w1160) -> ("States Out"=w1161:string)  [unwired: 14 in]
      }
      frame "MCLB: Reorder" {
        # "Multicolumn Listbox\n(You can make a copy of, or modify, this frame)"
        n448 = Unbundle By Name(w1171) -> ("MCLB"=w1169:refnum<class "Selector.lvclass">, "Item Names"=w1163:string[][])
        n449 = call-dynamic "Read Items.vi"("Selector in"=w1169) -> ("Items"=w1168:T33, "Selector out"=w1167:refnum<class "Selector.lvclass">)  [unwired: 8 in, 1 out]
        n450 = Index Array(array=w1163, index (col)=0 ("disabled index (col)")) -> (element=w1162:string[])  [unwired: 1 in]
        n451 = call "Items to Names.vi"("Items"=w1168) -> ("Names"=w1170:string[])  [unwired: 6 in]
        n452 = for {
          tunnel: w1168 -> [w1179]
          tunnel: w1170 -> [w1181]
          tunnel: w1162 -> [w1180] mode=indexing
          tunnel: [w1177] -> w1165 mode=indexing
          n453 = Search 1D Array(1D array=w1181, element=w1180) -> (index of element=w1178:i32)  [unwired: 1 in]
          n454 = Index Array(array=w1179, index=w1178) -> (element=w1177:T10)
        }
        n455 = call-dynamic "Write Items.vi"("Items"=w1165, "Selector in"=w1167) -> ("Selector out"=w1166:refnum<class "Selector.lvclass">)  [unwired: 8 in, 1 out]
        n456 = Bundle By Name(cluster=w1171, "MCLB"=w1166) -> (w1172:T20)
        n457 = call <vilib>:"Add State(s) to Queue__jki_lib_state_machine.vi"("State(s) in (\"\")"=w1174) -> ("States Out"=w1175:string)  [unwired: 14 in]
      }
      frame "MCLB: SCM Selection" {
        # "Multicolumn Listbox\n(You can make a copy of, or modify, this frame)"
        n458 = Unbundle By Name(w1185) -> ("Database"=w1184:refnum<class "Setting Database.lvclass">, "MCLB"=w1183:refnum<class "Selector.lvclass">)  [unwired: 1 out]
        n459 = Bundle By Name(cluster=w1185, "Database"=w1184, "MCLB"=w1183) -> (w1186:T20)
        n460 = call <vilib>:"Add State(s) to Queue__jki_lib_state_machine.vi"("State(s) in (\"\")"=w1188) -> ("States Out"=w1189:string)  [unwired: 14 in]
      }
      frame "MCLB: Populate New" {
        # "Multicolumn Listbox\n(You can make a copy of, or modify, this frame)"
        n461 = Unbundle By Name(w1191) -> ("MCLB"=w1190:refnum<class "Selector.lvclass">)
        n462 = Bundle By Name(cluster=w1191, "MCLB"=w1190) -> (w1192:T20)
        n463 = call <vilib>:"Add State(s) to Queue__jki_lib_state_machine.vi"("State(s) in (\"\")"=w1194) -> ("States Out"=w1195:string)  [unwired: 14 in]
      }
      frame "MCLB: Generate Names" {
        # "Multicolumn Listbox\n(You can make a copy of, or modify, this frame)"
        n464 = Unbundle By Name(w1214) -> ("MCLB"=w1205:refnum<class "Selector.lvclass">, "Tooler"=w1213:refnum<class "Tool Data.lvclass">, "IDs.paths"=w1212:string[], "IDs.funnels"=w1211:string[], "IDs.rects"=w1210:string[], "IDs.dots"=w1209:string[])
        n465 = Array Size(array=w1211) -> (size(s)=w1199:i32)
        n466 = Array Size(array=w1212) -> (size(s)=w1200:i32)
        n467 = Array Size(array=w1210) -> (size(s)=w1198:i32)
        n468 = Array Size(array=w1209) -> (size(s)=w1197:i32)
        n469 = Build Array(w1200, w1199, w1198, w1197) -> (w1208:i32[])
        n470 = for {
          tunnel: w1208 -> [w1220] mode=indexing
          tunnel: string[] ["p", "f", "r", "d"] -> [w1222] mode=indexing
          tunnel: [w1221] -> w1202 mode=concatenating
          n471 = for {
            N: w1220 -> [_]
            tunnel: w1222 -> [w1227]
            tunnel: [w1223] -> w1221 mode=indexing
            i -> [w1228]
            n472 = Number To Decimal String(number=w1228) -> (decimal integer string=w1226:string)  [unwired: 1 in]
            n473 = Concatenate Strings(w1227, w1226) -> (w1224:string)
            n474 = Bundle By Name(cluster=T10 {"Name"="", "Group"="", "Enabled"=FALSE} ("element"), "Name"=w1224) -> (w1223:T10)
          }
        }
        n475 = call-dynamic "Read Reference.vi"("Selector in"=w1205) -> ("Reference"=w1203:refnum<vi>, "Selector out"=w1204:refnum<class "Selector.lvclass">)  [unwired: 8 in, 1 out]
        n476 = call "Items to MCLB Item Names.vi"("Items"=w1202) -> ("Item Names"=w1201:string[][])  [unwired: 6 in]
        n477 = call-dynamic "Write Items.vi"("Items"=w1202, "Selector in"=w1204) -> ("Selector out"=w1206:refnum<class "Selector.lvclass">)  [unwired: 8 in, 1 out]
        n478 = property class="MCListbox"(reference=w1203, "ItemNames"=w1201) -> ()  [unwired: 1 in, 2 out]
        n479 = Bundle By Name(cluster=w1214, "MCLB"=w1206, "Tooler"=w1213) -> (w1215:T20)
        n480 = call <vilib>:"Add State(s) to Queue__jki_lib_state_machine.vi"("State(s) in (\"\")"=w1217) -> ("States Out"=w1218:string)  [unwired: 14 in]
      }
      frame "---------- Configuration ----------" {
        # "Template Separator\n(You can make a copy of, or modify, this frame)"
        n481 = Unbundle By Name(w1230) -> ("Background Image"=w1229:path)
        n482 = Bundle By Name(cluster=w1230, "Background Image"=w1229) -> (w1231:T20)
        n483 = call <vilib>:"Add State(s) to Queue__jki_lib_state_machine.vi"("State(s) in (\"\")"=w1233) -> ("States Out"=w1234:string)  [unwired: 14 in]
      }
      frame "Configuration: Write" {
        # "Write new information to the configuration file for next time we use program"
        n484 = Unbundle By Name(w1247) -> ("Config"=w1236:refnum<class "Configuration.lvclass">, "Inkscape File (.svg)"=w1245:path, "Background Image"=w1244:path, "Autosave Path"=w1243:path, "Autosave?"=w1242:bool)
        n485 = Bundle(cluster=T11 {"Inkscape Path"=path "", "Background Path"=path "", "Autosave Render Path"=path "", "Autosave Render"=FALSE} ("Configuration Data"), "Inkscape Path"=w1245, "Background Path"=w1244, "Autosave Render Path"=w1243, "Autosave Render"=w1242) -> (w1237:T11)
        n486 = call <userlib>:"Write Configuration.vi"("error in (no error)"=w1239, "Variant"=w1237, "Configuration in"=w1236) -> ("error out"=w1238:errorcluster, "Configuration out"=w1240:refnum<class "Configuration.lvclass">)  [unwired: 7 in]
        n487 = Bundle By Name(cluster=w1247, "Config"=w1240) -> (w1248:T20)
        n488 = call <vilib>:"Add State(s) to Queue__jki_lib_state_machine.vi"("State(s) in Front (\"\")"="UI: Status >> Configuration Written" ("State(s) in Front (\"\")"), "State(s) in (\"\")"=w1250) -> ("States Out"=w1251:string)  [unwired: 13 in]
      }
      frame "Configuration: Read" {
        w1260 = T11 {"Inkscape Path"=path "", "Background Path"=path "", "Autosave Render Path"=path "", "Autosave Render"=FALSE} ("Configuration Data")
        # "Read Configuration Data from File"
        n489 = Unbundle By Name(w1265) -> ("Config"=w1264:refnum<class "Configuration.lvclass">)
        n490 = call <userlib>:"Read Configuration.vi"("INI Fomatted Cluster Type"=w1260, "error in (no error)"=w1262, "Configuration in"=w1264) -> ("error out"=w1258:errorcluster, "Configuration"=w1261:variant, "Configuration out"=w1263:refnum<class "Configuration.lvclass">)  [unwired: 6 in]
        n491 = Variant To Data(error in=w1258, type=w1260, Variant=w1261) -> (data=w1259:T11, error out=w1257:errorcluster)
        n492 = Unbundle(w1259) -> ("Inkscape Path"=w1256:path, "Background Path"=w1254:path, "Autosave Render Path"=w1253:path, "Autosave Render"=w1252:bool)
        n493 = Bundle By Name(cluster=w1265, "Config"=w1263, "Inkscape File (.svg)"=w1256, "Background Image"=w1254, "Autosave Path"=w1253, "Autosave?"=w1252) -> (w1266:T20)
        n494 = call <vilib>:"Add State(s) to Queue__jki_lib_state_machine.vi"("State(s) in Front (\"\")"="UI: Status >> Configuration Read\nUI: Background Path\nUI: Inkscape Path\nUI: Autosave Render Path", "State(s) in (\"\")"=w1268) -> ("States Out"=w1269:string)  [unwired: 13 in]
      }
      frame "Configuration: Initialize" {
        # "Initialize Configuration Class with Path to File"
        n495 = Unbundle By Name(w1277) -> ("Config"=w1276:refnum<class "Configuration.lvclass">)
        n496 = call "Base INI Folder Path.vi"() -> ("Base Path"=w1271:path)  [unwired: 11 in]
        n497 = call <userlib>:"Write Path.vi"("error in (no error)"=w1273, "Filename [Configuration.ini]"="Config.ini" ("File (Configuration.ini)"), "Path"=w1271, "Configuration in"=w1276) -> ("error out"=w1274:errorcluster, "Configuration out"=w1275:refnum<class "Configuration.lvclass">)  [unwired: 6 in]
        n498 = Bundle By Name(cluster=w1277, "Config"=w1275) -> (w1278:T20)
        n499 = call <vilib>:"Add State(s) to Queue__jki_lib_state_machine.vi"("State(s) in Front (\"\")"="UI: Status >> Configuration Initialized" ("State(s) in Front (\"\")"), "State(s) in (\"\")"=w1280) -> ("States Out"=w1281:string)  [unwired: 13 in]
      }
      frame "---------- Driver ----------" {
        # "Template Separator\n(You can make a copy of, or modify, this frame)"
        n500 = call <vilib>:"Add State(s) to Queue__jki_lib_state_machine.vi"("State(s) in (\"\")"=w1283) -> ("States Out"=w1285:string)  [unwired: 14 in]
      }
      frame "Driver: Init Manager" {
        # "Template Separator\n(You can make a copy of, or modify, this frame)"
        n501 = Unbundle By Name(w1288) -> ("AFM_Driver_Manager"=w1293:refnum<class "AFM_Driver_Manager.lvclass">)
        n502 = call "AFM_Driver_Manager.Initialize.vi"("error in (no error)"=w1289, "AFM_Driver_Manager in"=w1293) -> ("error out"=w1290:errorcluster, "AFM_Driver_Manager out"=w1291:refnum<class "AFM_Driver_Manager.lvclass">)  [unwired: 8 in]
        n503 = Bundle By Name(cluster=w1288, "AFM_Driver_Manager"=w1291) -> (w1292:T20)
        n504 = call <vilib>:"Add State(s) to Queue__jki_lib_state_machine.vi"("State(s) in Front (\"\")"="UI: Status >> AFM Driver Manager Initialized" ("State(s) in Front (\"\")"), "State(s) in (\"\")"=w1295) -> ("States Out"=w1296:string)  [unwired: 13 in]
      }
      frame "Driver: Init Drivers" {
        # "Initialized an AFM_Driver_Manager Class using paths to the drivers.\n(All drivers will be started.)"
        n505 = Unbundle By Name(w1299) -> ("root path"=w1298:path)
        n506 = Unbundle By Name(w1299) -> ("AFM_Driver_Manager"=w1300:refnum<class "AFM_Driver_Manager.lvclass">)
        n507 = Build Path(base path=w1298, name or relative path="AFMs\\Asylum_Driver\\Asylum_Driver.vi") -> (appended path=w1304:path)
        n508 = Build Array(w1304) -> (w1303:path[])
        n509 = call "AFM_Driver_Manager.InitializeDrivers.vi"("error in (no error)"=w1307, "Paths"=w1303, "AFM_Driver_Manager in"=w1300) -> ("error out"=w1308:errorcluster, "AFM_Driver_Manager out"=w1305:refnum<class "AFM_Driver_Manager.lvclass">)  [unwired: 7 in]
        n510 = Bundle By Name(cluster=w1299, "AFM_Driver_Manager"=w1305) -> (w1306:T20)
        n511 = call <vilib>:"Add State(s) to Queue__jki_lib_state_machine.vi"("State(s) in Front (\"\")"="UI: Status >> AFM Driver Initialized" ("State(s) in Front (\"\")"), "State(s) in (\"\")"=w1309) -> ("States Out"=w1310:string)  [unwired: 13 in]
      }
      frame "Driver: Set Active" {
        # "Change the Active Driver. Call this state as Driver: Set Active >> # \n(where # is the panel to set active)"
        n512 = Decimal String To Number(string=w1313) -> (number=w1312:i32)  [unwired: 2 in, 1 out]
        n513 = Unbundle By Name(w1318) -> ("AFM_Driver_Manager"=w1317:refnum<class "AFM_Driver_Manager.lvclass">)
        n514 = call "AFM_Driver_Manager.SetActive.vi"("error in (no error)"=w1315, "Active Index"=w1312, "AFM_Driver_Manager in"=w1317) -> ("error out"=w1316:errorcluster, "AFM_Driver_Manager out"=w1319:refnum<class "AFM_Driver_Manager.lvclass">)  [unwired: 7 in]
        n515 = Bundle By Name(cluster=w1318, "AFM_Driver_Manager"=w1319) -> (w1320:T20)
        n516 = call <vilib>:"Add State(s) to Queue__jki_lib_state_machine.vi"("State(s) in Front (\"\")"="UI: Status >> Active Driver Selected" ("State(s) in Front (\"\")"), "State(s) in (\"\")"=w1321) -> ("States Out"=w1322:string)  [unwired: 13 in]
      }
      frame "Driver: Insert Into Subpanel" {
        # "Insert the Active Driver into the Subpanel provided\n(Active is by default panel 0)"
        n517 = Unbundle By Name(w1329) -> ("AFM_Driver_Manager"=w1331:refnum<class "AFM_Driver_Manager.lvclass">)
        n518 = control-ref of="AFM Settings"() -> (w1325:refnum<vi>)
        n519 = call "AFM_Driver_Manager.InsertActiveIntoSubpanel.vi"("error in (no error)"=w1326, "SubPnl Refnum"=w1325, "AFM_Driver_Manager in"=w1331) -> ("error out"=w1327:errorcluster, "AFM_Driver_Manager out"=w1328:refnum<class "AFM_Driver_Manager.lvclass">)  [unwired: 7 in]
        n520 = Bundle By Name(cluster=w1329, "AFM_Driver_Manager"=w1328) -> (w1330:T20)
        n521 = call <vilib>:"Add State(s) to Queue__jki_lib_state_machine.vi"("State(s) in Front (\"\")"="UI: Status >> AFM Driver inserted into subpanel" ("State(s) in Front (\"\")"), "State(s) in (\"\")"=w1332) -> ("States Out"=w1333:string)  [unwired: 13 in]
      }
      frame "Driver: Run Lithography" {
        # "Send a Command to the Driver to Run Lithography\n(You can make a copy of, or modify, this frame)"
        n522 = Unbundle By Name(w1337) -> ("AFM_Driver_Manager"=w1341:refnum<class "AFM_Driver_Manager.lvclass">)
        n523 = call "AFM_Driver_Manager.SendRun.vi"("error in (no error)"=w1339, "AFM_Driver_Manager in"=w1341) -> ("error out"=w1340:errorcluster, "AFM_Driver_Manager out"=w1336:refnum<class "AFM_Driver_Manager.lvclass">)  [unwired: 8 in]
        n524 = Bundle By Name(cluster=w1337, "AFM_Driver_Manager"=w1336) -> (w1338:T20)
        n525 = call <vilib>:"Add State(s) to Queue__jki_lib_state_machine.vi"("State(s) in Front (\"\")"="UI: Status >> Run Litho Msg Sent to Driver" ("State(s) in Front (\"\")"), "State(s) in (\"\")"=w1342) -> ("States Out"=w1343:string)  [unwired: 13 in]
      }
      frame "Driver: Litho Data" {
        # "Update the value of the lithography data in the driver\n(You can make a copy of, or modify, this frame)"
        n526 = Unbundle By Name(w1347) -> ("AFM_Driver_Manager"=w1351:refnum<class "AFM_Driver_Manager.lvclass">, "Lithography Data"=w1352:T27)
        n527 = call "AFM_Driver_Manager.SendLithography.vi"("error in (no error)"=w1344, "Lithography Data"=w1352, "AFM_Driver_Manager in"=w1351) -> ("error out"=w1345:errorcluster, "AFM_Driver_Manager out"=w1350:refnum<class "AFM_Driver_Manager.lvclass">)  [unwired: 7 in]
        n528 = Bundle By Name(cluster=w1347, "AFM_Driver_Manager"=w1350) -> (w1349:T20)
        n529 = call <vilib>:"Add State(s) to Queue__jki_lib_state_machine.vi"("State(s) in Front (\"\")"="UI: Status >> Lithography Data Sent to Driver" ("State(s) in Front (\"\")"), "State(s) in (\"\")"=w1353) -> ("States Out"=w1354:string)  [unwired: 13 in]
      }
      frame "Driver: Background Image" {
        # "Send the Background Image Path to the driver\n(You can make a copy of, or modify, this frame)"
        n530 = Unbundle By Name(w1357) -> ("AFM_Driver_Manager"=w1363:refnum<class "AFM_Driver_Manager.lvclass">, "Background Image"=w1356:path)
        n531 = call "AFM_Driver_Manager.SendBackgroundImage.vi"("error in (no error)"=w1361, "Path"=w1356, "AFM_Driver_Manager in"=w1363) -> ("error out"=w1362:errorcluster, "AFM_Driver_Manager out"=w1359:refnum<class "AFM_Driver_Manager.lvclass">)  [unwired: 7 in]
        n532 = Bundle By Name(cluster=w1357, "AFM_Driver_Manager"=w1359) -> (w1360:T20)
        n533 = call <vilib>:"Add State(s) to Queue__jki_lib_state_machine.vi"("State(s) in Front (\"\")"="UI: Status >> Background Image Sent to Driver" ("State(s) in Front (\"\")"), "State(s) in (\"\")"=w1364) -> ("States Out"=w1365:string)  [unwired: 13 in]
      }
      frame "Driver: Stop Manager" {
        # "Stops all drivers.\n(You can make a copy of, or modify, this frame)"
        n534 = Unbundle By Name(w1371) -> ("AFM_Driver_Manager"=w1370:refnum<class "AFM_Driver_Manager.lvclass">)
        n535 = call "AFM_Driver_Manager.Shutdown.vi"("error in (no error)"=w1368, "AFM_Driver_Manager in"=w1370) -> ("error out"=w1369:errorcluster)  [unwired: 9 in]
        n536 = call <vilib>:"Add State(s) to Queue__jki_lib_state_machine.vi"("State(s) in Front (\"\")"="UI: Status >> AFM Driver Manager Shut Down" ("State(s) in Front (\"\")"), "State(s) in (\"\")"=w1372) -> ("States Out"=w1373:string)  [unwired: 13 in]
      }
      frame "---------- Parser ----------" {
        # "Template Separator\n(You can make a copy of, or modify, this frame)"
        n537 = Unbundle By Name(w1375) -> ("ParseVectorFile"=w1374:refnum<class "ParseVectorFile.lvclass">)
        n538 = Bundle By Name(cluster=w1375, "ParseVectorFile"=w1374) -> (w1376:T20)
        n539 = call <vilib>:"Add State(s) to Queue__jki_lib_state_machine.vi"("State(s) in (\"\")"=w1378) -> ("States Out"=w1379:string)  [unwired: 14 in]
      }
      frame "Parser: Parse SVG" {
        # "New parser is about 1/2 the speed of old parser (~15 ms vs ~35 ms), but is better in almost every other aspect that actually counts"
        # "Parses an SVG file\n(You can make a copy of, or modify, this frame)"
        n540 = Unbundle By Name(w1408) -> ("Tooler"=w1404:refnum<class "Tool Data.lvclass">, "ParseVectorFile"=w1406:refnum<class "ParseVectorFile.lvclass">, "Inkscape File (.svg)"=w1407:path)
        n541 = call "ParseVectorFile.NewFileSynchronous.vi"("timeout in ms (-1)"=20000, "error in (no error)"=w1384, "Path"=w1407, "ParseVectorFile"=w1406) -> ("error out"=w1382:errorcluster, "ParsedData"=w1400:T34, "ParseVectorFile out"=w1390:refnum<class "ParseVectorFile.lvclass">)  [unwired: 5 in]
        n542 = Unbundle By Name(w1400) -> ("Paths"=w1399:refnum<class "Path.lvclass">[], "Rectangles"=w1398:refnum<class "Rectangle.lvclass">[], "SVGImage"=w1383:refnum<class "SVGImage.lvclass">, "Dots"=w1397:refnum<class "Dot.lvclass">[])
        n543 = call-dynamic "Read Data.vi"("error in (no error)"=w1382, "Tool Data in"=w1404) -> ("error out"=w1381:errorcluster, "Data"=w1402:T35, "Tool Data out"=w1403:refnum<class "Tool Data.lvclass">)  [unwired: 7 in]
        n544 = property class="SVGImage.lvclass"(reference=w1383) -> ("Accessors:Height"=w1387:dbl, "Accessors:Width"=w1386:dbl)  [unwired: 1 in, 2 out]
        n545 = Bundle By Name(cluster=w1402, "Paths"=w1399, "Rectangles"=w1398, "SVGImage"=w1383, "Dots"=w1397) -> (w1401:T35)
        n546 = call-dynamic "Write Data.vi"("error in (no error)"=w1381, "Data"=w1401, "Tool Data in"=w1403) -> ("error out"=w1396:errorcluster, "Tool Data out"=w1391:refnum<class "Tool Data.lvclass">)  [unwired: 7 in]
        n547 = Bundle By Name(cluster=cluster{"Width":dbl, "Height":dbl} {"Width"=0.0, "Height"=0.0} ("Image Size In"), "Height"=w1387, "Width"=w1386) -> (w1385:cluster{"Width":dbl, "Height":dbl})
        n548 = call "Sort Funnels and Paths.vi"("error in (no error)"=w1396, "Tool Data in"=w1391) -> ("error out"=w1394:errorcluster, "Tool Data out"=w1395:refnum<class "Tool Data.lvclass">)  [unwired: 8 in]
        n549 = call "Set Inkscape Ratio.vi"("Image Size In"=w1385) -> ("Image Size Out"=w1410:cluster{"Width":dbl, "Height":dbl})
        n550 = call "Get IDs.vi"("error in (no error)"=w1394, "Tool Data in"=w1395) -> ("error out"=w1393:errorcluster, "IDs"=w1392:T24)  [unwired: 7 in, 1 out]
        n551 = Bundle By Name(cluster=w1408, "Tooler"=w1391, "ParseVectorFile"=w1390, "IDs"=w1392) -> (w1409:T20)
        n552 = global write "Global Variables.vi" "Size"(w1410) -> ()
        n553 = call <vilib>:"Add State(s) to Queue__jki_lib_state_machine.vi"("State(s) in Front (\"\")"="UI: Status >> File parsed.\nMCLB: Generate Names" ("State(s) in Front (\"\")"), "State(s) in (\"\")"=w1412) -> ("States Out"=w1413:string)  [unwired: 13 in]
      }
      frame "Parser: Stop" {
        # "Template Separator\n(You can make a copy of, or modify, this frame)"
        n554 = Unbundle By Name(w1421) -> ("ParseVectorFile"=w1418:refnum<class "ParseVectorFile.lvclass">)
        n555 = call <vilib>:"Stop.vi"("error in (no error)"=w1416, "SMO"=w1418) -> ("error out"=w1419:errorcluster, "SMO out"=w1420:refnum<class "ParseVectorFile.lvclass">)  [unwired: 8 in]
        n556 = call <vilib>:"Destroy.vi"("error in (no error)"=w1419, "SMO"=w1420) -> ("error out"=w1417:errorcluster)  [unwired: 9 in]
        n557 = Bundle By Name(cluster=w1421, "ParseVectorFile"=refnum<class "ParseVectorFile.lvclass"> refnum) -> (w1422:T20)
        n558 = call <vilib>:"Add State(s) to Queue__jki_lib_state_machine.vi"("State(s) in Front (\"\")"="UI: Status >> Parser Stopped" ("State(s) in Front (\"\")"), "State(s) in (\"\")"=w1424) -> ("States Out"=w1425:string)  [unwired: 13 in]
      }
      frame "Parser: Start" {
        # "Template Separator\n(You can make a copy of, or modify, this frame)"
        n559 = Unbundle By Name(w1433) -> ("ParseVectorFile"=w1432:refnum<class "ParseVectorFile.lvclass">)
        n560 = call <vilib>:"Create.vi"("error in (no error)"=w1427, "SMO"=w1432) -> ("error out"=w1429:errorcluster, "SMO out"=w1431:refnum<class "ParseVectorFile.lvclass">)  [unwired: 7 in, 1 out]
        n561 = call <vilib>:"Start.vi"("error in (no error)"=w1429, "SMO"=w1431) -> ("error out"=w1428:errorcluster, "SMO out"=w1430:refnum<class "ParseVectorFile.lvclass">)  [unwired: 8 in]
        n562 = Bundle By Name(cluster=w1433, "ParseVectorFile"=w1430) -> (w1434:T20)
        n563 = call <vilib>:"Add State(s) to Queue__jki_lib_state_machine.vi"("State(s) in Front (\"\")"="UI: Status >> Parser started." ("State(s) in Front (\"\")"), "State(s) in (\"\")"=w1436) -> ("States Out"=w1437:string)  [unwired: 13 in]
      }
      frame "---------- Database ----------" {
        # "Template Separator\n(You can make a copy of, or modify, this frame)"
        n564 = Unbundle By Name(w1439) -> ("Database"=w1438:refnum<class "Setting Database.lvclass">)
        n565 = Bundle By Name(cluster=w1439, "Database"=w1438) -> (w1440:T20)
        n566 = call <vilib>:"Add State(s) to Queue__jki_lib_state_machine.vi"("State(s) in (\"\")"=w1442) -> ("States Out"=w1443:string)  [unwired: 14 in]
      }
      frame "Database: Update Enable" {
        # "Template Separator\n(You can make a copy of, or modify, this frame)"
        n567 = Unbundle By Name(w1450) -> ("Database"=w1449:refnum<class "Setting Database.lvclass">)
        n568 = call "Setting Database.ChangeObjectEnable.vi"("error in (no error)"=w1446, "ChangeObjectEnable"=w1445, "Setting Database"=w1449) -> ("error out"=w1447:errorcluster, "Setting Database out"=w1448:refnum<class "Setting Database.lvclass">)  [unwired: 7 in]
        n569 = Bundle By Name(cluster=w1450, "Database"=w1448) -> (w1451:T20)
        n570 = call <vilib>:"Add State(s) to Queue__jki_lib_state_machine.vi"("State(s) in (\"\")"=w1453) -> ("States Out"=w1454:string)  [unwired: 14 in]
      }
      frame "Database: Set Active" {
        # "Template Separator\n(You can make a copy of, or modify, this frame)"
        n571 = call "Name To Type.vi"("Name"=w1455) -> ("Type"=w1457:string)  [unwired: 4 in]
        n572 = call "Name To Index.vi"("Name"=w1455) -> ("Index"=w1456:i32)  [unwired: 4 in]
        n573 = Unbundle By Name(w1463) -> ("Database"=w1462:refnum<class "Setting Database.lvclass">)
        n574 = case shown="\"d\"" w1457 {
          tunnel: w1462 -> [w1472 w1474 w1479 w1484 w1489 w1493]
          tunnel: [w1471 w1473 w1478 w1482 w1487 w1492] -> w1461
          tunnel: w1460 -> [w1468 w1473 w1477 w1481 w1486 w1491]
          tunnel: [w1472 w1474 w1476 w1483 w1488 w1494] -> w1459
          tunnel: w1456 -> [_ _ w1475 w1480 w1485 w1490]
          frame Default {
            n575 = call <vilib>:"Error Cluster From Error Code.vi"("error in (no error)"=w1468, "error message (\"\")"="Unknown Object Type. Cannot Set Active In Database" ("error message (\"\")"), "error code (0)"=1) -> ("error out"=w1471:errorcluster)  [unwired: 6 in]
          }
          frame "" {
            # "There are no objects to set as active\n\nTemp fix for issue \\#78:\nhttps://github.com/levylabpitt/AFM-Lithography/issues/78"
          }
          frame "p" {
            n576 = call "Setting Database.SetActivePath.vi"("error in (no error)"=w1477, "SetActivePath"=w1475, "Setting Database"=w1479) -> ("error out"=w1478:errorcluster, "Setting Database out"=w1476:refnum<class "Setting Database.lvclass">)  [unwired: 7 in]
          }
          frame "r" {
            n577 = call "Setting Database.SetActiveRectangle.vi"("error in (no error)"=w1481, "SetActiveRectangle"=w1480, "Setting Database"=w1484) -> ("error out"=w1482:errorcluster, "Setting Database out"=w1483:refnum<class "Setting Database.lvclass">)  [unwired: 7 in]
          }
          frame "f" {
            n578 = call "Setting Database.SetActiveFunnel.vi"("error in (no error)"=w1486, "SetActiveFunnel"=w1485, "Setting Database"=w1489) -> ("error out"=w1487:errorcluster, "Setting Database out"=w1488:refnum<class "Setting Database.lvclass">)  [unwired: 7 in]
          }
          frame "d" {
            # "Need to send the data event here"
            n579 = call "Setting Database.SetActiveDot.vi"("error in (no error)"=w1491, "SetActiveDot"=w1490, "Setting Database"=w1493) -> ("error out"=w1492:errorcluster, "Setting Database out"=w1494:refnum<class "Setting Database.lvclass">)  [unwired: 7 in]
          }
        }
        n580 = Bundle By Name(cluster=w1463, "Database"=w1459) -> (w1464:T20)
        n581 = call <vilib>:"Add State(s) to Queue__jki_lib_state_machine.vi"("State(s) in Front (\"\")"="UI: Status >> Database: Active Object Set" ("State(s) in Front (\"\")"), "State(s) in (\"\")"=w1466) -> ("States Out"=w1467:string)  [unwired: 13 in]
      }
      frame "Database: Refresh" {
        # "This can be updated to have IDs, which will allow for more control over keeping settings"
        # "Handle UI changes to account for the fact that the active value is once again zero. I am treating it like a click (generating a UI Event with the signalling property) because I want to go through the logic as if it was identical to a user selecting a different value."
        # "Template Separator\n(You can make a copy of, or modify, this frame)"
        n582 = Unbundle By Name(w1510) -> ("Database"=w1509:refnum<class "Setting Database.lvclass">, "IDs.paths"=w1498:string[], "IDs.funnels"=w1497:string[], "IDs.rects"=w1496:string[], "IDs.dots"=w1495:string[])
        n583 = Bundle By Name(cluster=T12 {"Paths"=[], "Rectangles"=[], "Funnels"=[], "Dots"=[]} ("Initialize"), "Paths"=w1498, "Funnels"=w1497, "Rectangles"=w1496, "Dots"=w1495) -> (w1506:T12)
        n584 = call "Setting Database.Refresh.vi"("error in (no error)"=w1501, "Initialize"=w1506, "Setting Database"=w1509) -> ("error out"=w1503:errorcluster, "Setting Database out"=w1508:refnum<class "Setting Database.lvclass">)  [unwired: 7 in]
        n585 = control-ref of="Patterns"() -> (w1505:refnum<vi>)
        n586 = property class="LstBox (strict)"(reference=w1505, error in=w1503, "Val(Sgnl)"=0 ("Value")) -> (error out=w1500:errorcluster)  [unwired: 1 out]
        n587 = Bundle By Name(cluster=w1510, "Database"=w1508) -> (w1511:T20)
        n588 = Merge Errors(w1500) -> (w1499:errorcluster)
        n589 = call <vilib>:"Add State(s) to Queue__jki_lib_state_machine.vi"("State(s) in Front (\"\")"="UI: Status >> Database Refresh Msg Sent" ("State(s) in Front (\"\")"), "State(s) in (\"\")"=w1513) -> ("States Out"=w1514:string)  [unwired: 13 in]
      }
      frame "Database: Refresh Sync" {
        # "#issue\nThis might be the cause of the odd timing in the order data VI?"
        # "Template Separator\n(You can make a copy of, or modify, this frame)"
        n590 = Unbundle By Name(w1549) -> ("Database"=w1545:refnum<class "Setting Database.lvclass">, "IDs.paths"=w1533:string[], "IDs.funnels"=w1532:string[], "IDs.rects"=w1531:string[], "IDs.dots"=w1530:string[], "Tooler"=w1527:refnum<class "Tool Data.lvclass">)
        n591 = control-ref of="Patterns"() -> (w1547:refnum<vi>)
        n592 = property class="LstBox (strict)"(reference=w1547, error in=w1536, "Value"=0) -> (error out=w1535:errorcluster)  [unwired: 1 out]
        n593 = Bundle By Name(cluster=T12 {"Paths"=[], "Rectangles"=[], "Funnels"=[], "Dots"=[]} ("Initialize"), "Paths"=w1533, "Funnels"=w1532, "Rectangles"=w1531, "Dots"=w1530) -> (w1543:T12)
        n594 = Merge Errors(w1535) -> (w1534:errorcluster)
        n595 = call <userlib>:"Tick Count (ms)__ogtk.vi"("error in (no error)"=w1534) -> ("error out"=w1540:errorcluster, "millisecond timer value"=w1538:u32)  [unwired: 9 in]
        n596 = call "Setting Database.Refresh.Synchronous.vi"("Timeout"=-1, "error in (no error)"=w1540, "Initialize"=w1543, "Setting Database in"=w1545) -> ("error out"=w1518:errorcluster, "Response"=w1524:T21, "Setting Database out"=w1544:refnum<class "Setting Database.lvclass">)  [unwired: 5 in]
        n597 = Unbundle By Name(w1524) -> ("Paths"=w1523:T14, "Rectangles"=w1522:T15, "Funnels"=w1521:T16, "Dots"=w1520:T17)
        n598 = call-dynamic "Read Settings.vi"("error in (no error)"=w1518, "Tool Data in"=w1527) -> ("error out"=w1519:errorcluster, "Settings"=w1526:T21, "Tool Data out"=w1528:refnum<class "Tool Data.lvclass">)  [unwired: 7 in]
        n599 = Bundle By Name(cluster=w1526, "Paths"=w1523, "Rectangles"=w1522, "Funnels"=w1521, "Dots"=w1520) -> (w1525:T21)
        n600 = call <userlib>:"Tick Count (ms)__ogtk.vi"("error in (no error)"=w1518) -> ("error out"=w1517:errorcluster, "millisecond timer value"=w1539:u32)  [unwired: 9 in]
        n601 = call-dynamic "Write Settings.vi"("error in (no error)"=w1519, "Settings"=w1525, "Tool Data in"=w1528) -> ("error out"=w1516:errorcluster, "Tool Data out"=w1529:refnum<class "Tool Data.lvclass">)  [unwired: 7 in]
        n602 = Subtract(x=w1539, y=w1538) -> ()  [unwired: 1 out]
        n603 = Bundle By Name(cluster=w1549, "Database"=w1544, "Tooler"=w1529) -> (w1550:T20)
        n604 = Merge Errors(w1516, w1517) -> (w1515:errorcluster)
        n605 = call <vilib>:"Add State(s) to Queue__jki_lib_state_machine.vi"("State(s) in Front (\"\")"="UI: Status >> Database Refreshed (Sync)" ("State(s) in Front (\"\")"), "State(s) in (\"\")"=w1552, "State(s) at Back (\"\")"="UI: Status >> New Active Object Selected\nMCLB: Symbols\nUI: Update Subpanel\nLitho: Order Data\nDriver: Litho Data" ("State(s) at Back (\"\")")) -> ("States Out"=w1553:string)  [unwired: 12 in]
      }
      frame "Database: Start" {
        # "Shared resource"
        # "This needs to be called before the Path Edit is started, otherwise path edit wont be able to find the shared resource"
        # "Template Separator\n(You can make a copy of, or modify, this frame)"
        n606 = Unbundle By Name(w1564) -> ("Database"=w1559:refnum<class "Setting Database.lvclass">)
        n607 = call "Setting Database Name.vi"("error in (no error)"=w1555) -> ("error out"=w1556:errorcluster, "Name"=w1561:string)  [unwired: 9 in]
        n608 = call <vilib>:"Create.vi"("Shared Resource (F)"=TRUE, "error in (no error)"=w1556, "Subsystem Name (optional)"=w1561, "SMO"=w1559) -> ("error out"=w1560:errorcluster, "SMO out"=w1563:refnum<class "Setting Database.lvclass">)  [unwired: 5 in, 1 out]
        n609 = call <vilib>:"Start.vi"("error in (no error)"=w1560, "SMO"=w1563) -> ("error out"=w1557:errorcluster, "SMO out"=w1558:refnum<class "Setting Database.lvclass">)  [unwired: 8 in]
        n610 = Bundle By Name(cluster=w1564, "Database"=w1558) -> (w1565:T20)
        n611 = call <vilib>:"Add State(s) to Queue__jki_lib_state_machine.vi"("State(s) in Front (\"\")"="UI: Status >> Settings Database Started" ("State(s) in Front (\"\")"), "State(s) in (\"\")"=w1567) -> ("States Out"=w1568:string)  [unwired: 13 in]
      }
      frame "Database: Stop" {
        # "Only call this on shutdown, otherwise it might cause problems with shared resource."
        # "Template Separator\n(You can make a copy of, or modify, this frame)"
        n612 = Unbundle By Name(w1576) -> ("Database"=w1574:refnum<class "Setting Database.lvclass">)
        n613 = call <vilib>:"Stop.vi"("error in (no error)"=w1570, "SMO"=w1574) -> ("error out"=w1572:errorcluster, "SMO out"=w1573:refnum<class "Setting Database.lvclass">)  [unwired: 8 in]
        n614 = call <vilib>:"Destroy.vi"("error in (no error)"=w1572, "SMO"=w1573) -> ("error out"=w1571:errorcluster)  [unwired: 9 in]
        n615 = Bundle By Name(cluster=w1576, "Database"=refnum<class "Setting Database.lvclass"> refnum) -> (w1577:T20)
        n616 = call <vilib>:"Add State(s) to Queue__jki_lib_state_machine.vi"("State(s) in Front (\"\")"="UI: Status >> Settings Database Stopped" ("State(s) in Front (\"\")"), "State(s) in (\"\")"=w1579) -> ("States Out"=w1580:string)  [unwired: 13 in]
      }
      frame "---------- Tooler ----------" {
        # "Template Separator\n(You can make a copy of, or modify, this frame)"
        n617 = Unbundle By Name(w1583) -> ("Tooler"=w1581:refnum<class "Tool Data.lvclass">)
        n618 = Bundle By Name(cluster=w1583, "Tooler"=w1581) -> (w1584:T20)
        n619 = call <vilib>:"Add State(s) to Queue__jki_lib_state_machine.vi"("State(s) in (\"\")"=w1586) -> ("States Out"=w1587:string)  [unwired: 14 in]
      }
      frame "Tooler: Stop" {
        # "Template Separator\n(You can make a copy of, or modify, this frame)"
        n620 = Unbundle By Name(w1594) -> ("Tooler"=w1593:refnum<class "Tool Data.lvclass">)
        n621 = call <vilib>:"Stop.vi"("error in (no error)"=w1588, "SMO"=w1593) -> ("error out"=w1590:errorcluster, "SMO out"=w1592:refnum<class "Tool Data.lvclass">)  [unwired: 8 in]
        n622 = call <vilib>:"Destroy.vi"("error in (no error)"=w1590, "SMO"=w1592) -> ("error out"=w1589:errorcluster)  [unwired: 9 in]
        n623 = Bundle By Name(cluster=w1594, "Tooler"=refnum<class "Tool Data.lvclass"> refnum) -> (w1595:T20)
        n624 = call <vilib>:"Add State(s) to Queue__jki_lib_state_machine.vi"("State(s) in (\"\")"=w1597) -> ("States Out"=w1598:string)  [unwired: 14 in]
      }
      frame "Tooler: Start" {
        # "Template Separator\n(You can make a copy of, or modify, this frame)"
        n625 = Unbundle By Name(w1605) -> ("Tooler"=w1602:refnum<class "Tool Data.lvclass">)
        n626 = call <vilib>:"Create.vi"("error in (no error)"=w1599, "SMO"=w1602) -> ("error out"=w1604:errorcluster, "SMO out"=w1603:refnum<class "Tool Data.lvclass">)  [unwired: 7 in, 1 out]
        n627 = call <vilib>:"Start.vi"("error in (no error)"=w1604, "SMO"=w1603) -> ("error out"=w1600:errorcluster, "SMO out"=w1601:refnum<class "Tool Data.lvclass">)  [unwired: 8 in]
        n628 = Bundle By Name(cluster=w1605, "Tooler"=w1601) -> (w1606:T20)
        n629 = call <vilib>:"Add State(s) to Queue__jki_lib_state_machine.vi"("State(s) in (\"\")"=w1608) -> ("States Out"=w1609:string)  [unwired: 14 in]
      }
      frame "Tooler: Objects" {
        # "Template Separator\n(You can make a copy of, or modify, this frame)"
        n630 = Unbundle By Name(w1635) -> ("Tooler"=w1633:refnum<class "Tool Data.lvclass">)
        n631 = call-dynamic "Read Data.vi"("error in (no error)"=w1624, "Tool Data in"=w1633) -> ("error out"=w1625:errorcluster, "Data"=w1627:T35, "Tool Data out"=w1632:refnum<class "Tool Data.lvclass">)  [unwired: 7 in]
        n632 = call-dynamic "Read Settings.vi"("error in (no error)"=w1625, "Tool Data in"=w1632) -> ("error out"=w1626:errorcluster, "Settings"=w1628:T21, "Tool Data out"=w1631:refnum<class "Tool Data.lvclass">)  [unwired: 7 in]
        n633 = Bundle By Name(cluster=T13 {"Settings"={"Paths"=[], "Rectangles"=[], "Funnels"=[], "Dots"=[]}, "Data"={"Paths"=[], "Rectangles"=[], "SVGImage"=refnum, "Dots"=[], "Funnels"=[]}} ("Update Objects"), "Settings"=w1628, "Data"=w1627) -> (w1629:T13)
        n634 = call-dynamic "Tool Data.ToolObjectsSynchronous.vi"("Timeout"=20000, "error in (no error)"=w1626, "Update Objects"=w1629, "Tool Data in"=w1631) -> ("error out"=w1619:errorcluster, "Object Updated"=w1617:T36, "Tool Data out"=w1621:refnum<class "Tool Data.lvclass">)  [unwired: 5 in]
        n635 = call-dynamic "Write Tooled.vi"("error in (no error)"=w1619, "Tooled"=w1617, "Tool Data in"=w1621) -> ("error out"=w1618:errorcluster, "Tool Data out"=w1620:refnum<class "Tool Data.lvclass">)  [unwired: 7 in]
        n636 = call-dynamic "Generate Lithography Data.vi"("error in (no error)"=w1618, "Tool Data in"=w1620) -> ("error out"=w1622:errorcluster, "Lithography Data"=w1610:T27, "Tool Data out"=w1623:refnum<class "Tool Data.lvclass">)  [unwired: 7 in]
        n637 = call "Estimated Time Required.vi"("Lithography Data"=w1610) -> ("Estimated Time Required"=w1615:timestamp)
        n638 = for {
          tunnel: w1610 -> [w1641] mode=indexing
          tunnel: [w1640] -> w1611 mode=indexing
          n639 = Unbundle By Name(w1641) -> ("Name"=w1640:string)
        }
        n640 = Format Date/Time String(time format string (%c)="%H:%M:%S", seconds (now)=w1615) -> (date/time string=w1614:string)  [unwired: 1 in]
        n641 = Bundle By Name(cluster=w1635, "Tooler"=w1623, "Lithography Data"=w1610, "Drag and Drop.Working"=w1611) -> (w1636:T20)
        n642 = call <vilib>:"Build State String with Arguments__JKI_lib_State_Machine.vi"("Arguments (\"\")"=w1614, "State"="UI: Update Time") -> ("State with Arguments"=w1612:string)  [unwired: 4 in]
        n643 = call <vilib>:"Add State(s) to Queue__jki_lib_state_machine.vi"("State(s) in Front (\"\")"=w1612, "State(s) in (\"\")"=w1638) -> ("States Out"=w1639:string)  [unwired: 13 in]
      }
    }
    n644 = call <userlib>:"Tick Count (ms)__ogtk.vi"("error in (no error)"=w20) -> ("error out"=w17:errorcluster, "millisecond timer value"=w15:u32)  [unwired: 9 in]
    n645 = Subtract(x=w15, y=w14) -> (x-y=w13:u32)
  }
  n646 = for {
    tunnel: w4 -> [w1645] mode=indexing
    tunnel: w3 -> [w1646] mode=indexing
    tunnel: [w1642] -> w1 mode=indexing
    n647 = Number To Decimal String(number=w1646) -> (decimal integer string=w1643:string)  [unwired: 1 in]
    n648 = Concatenate Strings(w1645, "     " ("string"), w1643) -> (w1642:string)
  }
  n649 = control-ref of="Listbox"() -> (w2:refnum<vi>)
  n650 = property class="LstBox (strict)"(reference=w2, "Item Names"=w1) -> ()  [unwired: 1 in, 2 out]
